vi "Interface_main.vi"() -> ()   [LabVIEW 2013]
uses:
  Controls/Steering Inputs.ctl
  Controls/Intuitive Steering.ctl
  Controls/Steering Mode.ctl
  Controls/SpaceMouse_Parameters.ctl
  Controls/SpaceMouse_Buttons.ctl
  Controls/Fin Arrangement.ctl
  Controls/Swimbladder Tuning Parameters.ctl
  Controls/Sensors State.ctl
  Controls/Sepios General Parameters.ctl
  Controls/Fin Status.ctl
  myRIO/Sensors/IMU/IMU_Data_Type_Def.ctl
  Controls/Advanced Swimbladder Indicators.ctl
  Controls/Battery_level.ctl
  Controls/Sepios_status.ctl
  Controls/Attitude Controllers Parameters.ctl
  Controls/EKF_Settings.ctl
  Controls/Estimated Position.ctl
  Controls/Individual Steering.ctl
  Controls/IndividualSteering_f(x)_enum.ctl
  Controls/Flow/Flow_Velocity.ctl
  Controls/Flow/Flow_Acceleration.ctl
  Controls/Flow/Flow_Number_dig.ctl
  Controls/Individual Steering Configurations.ctl
  Controls/Flow/Flow_Throttle.ctl
  Controls/Flow/Velocity Controllers Parameters.ctl
  Controls/Flow/Flow_Variables.ctl
  Controls/SpaceMouse_FilteredInput.ctl
  Controls/SpaceMouse_RawInput.ctl
  Controls/Servo Position.ctl
  <vilib>/Utility/xml.llb/Write to XML File(string).vi
  <vilib>/Utility/xml.llb/Read From XML File(string).vi
  myRIO/Sensors/IMU/Attitude display/Bsp. Attitude Display/lv-attitudecontrol.lvlib
panel:
  out "Fin Status":T1=[16777215, 16777215, 16777215, 16777215]
  in  "Fin Arrangement":T2={"Fin0"=0, "Fin3"=3, "Fin1"=1, "Fin2"=2} {"Fin2" items=["0", "1", "2", "3"]; "Fin1" items=["0", "1", "2", "3"]; "Fin3" items=["0", "1", "2", "3"]; "Fin0" items=["0", "1", "2", "3"]}
  out "Main_Current [A]":dbl(knob) scale=0.0..50.0
  out "tooDeep":bool
  out "LEAKAGE":bool
  out "Depth [m]":cluster{dbl, dbl, dbl}(slide)={0.0, 0.0, 3.5} scale format="%#_3g"
  in  "Steering Mode":T3
  in  "Tab Control":T4(tab)
  in  "Attitude Sepios":refnum<vi>(3d-picture)
  out "Battery_level":T5=86.537845 scale=0.0..100.0
  in  "Full Battery?":bool
  out "Time left [min]":dbl=inf
  out "Sepios_Status":T6
  in  "Desired Attitude":refnum<vi>(3d-picture)
  in  "Attitude Control On":bool
  in  "Auto stable when idle":bool
  out "Brake":bool
  in  "STOP_Steering":bool
  in  "Intuitive Steering User Control":T7={"Frequency (Hz):"=0.7, "Max. Amplitude (°):"=25.0, "Phase Shift (/Pi):"=0.25, "Flap (°):"=90.0, "Flap Saturation:"=0.7} {"Flap Saturation:" min=0.0 max=1.0 step=0.1; "Flap (°):" min=0.0 max=90.0 step=5.0; "Phase Shift (/Pi):" min=-1.0 max=1.0 step=0.1; "Max. Amplitude (°):" min=0.0 max=135.0 step=1.0; "Frequency (Hz):" min=0.0 max=2.0 step=0.1}
  out "Bottom Fin (2)":cluster{dbl, dbl, "FinPositions":dbl[]}(graph)={0.0, 1.0, "FinPositions"=[0.0, 0.0, 0.0, 0.0, 0.0, 0.0, 0.0, 0.0, 0.0]}
  out "Right Fin (1)":cluster{dbl, dbl, "FinPositions":dbl[]}(graph)={0.0, 1.0, "FinPositions"=[0.0, 0.0, 0.0, 0.0, 0.0, 0.0, 0.0, 0.0, 0.0]}
  out "Left Fin (3)":cluster{dbl, dbl, "FinPositions":dbl[]}(graph)={0.0, 1.0, "FinPositions"=[0.0, 0.0, 0.0, 0.0, 0.0, 0.0, 0.0, 0.0, 0.0]}
  out "Top Fin (0)":cluster{dbl, dbl, "FinPositions":dbl[]}(graph)={0.0, 1.0, "FinPositions"=[0.0, 0.0, 0.0, 0.0, 0.0, 0.0, 0.0, 0.0, 0.0]}
  in  "IndividualSteering_f(x)":T8
  in  "Individual Steering":T9=[{"Fin Parameters"=[{"Amplitude"=20.0, "Phase Shift"=0.25, "Zero Position"=0.0}, {"Amplitude"=20.0, "Phase Shift"=0.25, "Zero Position"=0.0}, {"Amplitude"=20.0, "Phase Shift"=0.25, "Zero Position"=0.0}, {"Amplitude"=20.0, "Phase Shift"=0.25, "Zero Position"=0.0}, {"Amplitude"=20.0, "Phase Shift"=0.25, "Zero Position"=0.0}, {"Amplitude"=20.0, "Phase Shift"=0.25, "Zero Position"=0.0}, {"Amplitude"=20.0, "Phase Shift"=0.25, "Zero Position"=0.0}, {"Amplitude"=20.0, "Phase Shift"=0.25, "Zero Position"=0.0}, {"Amplitude"=20.0, "Phase Shift"=0.25, "Zero Position"=0.0}], "Frequency\n& Direction"=0.7, "General A, PS, ZP"={"Amplitude"=20.0, "Phase Shift"=0.25, "Zero Position"=0.0}}, {"Fin Parameters"=[{"Amplitude"=20.0, "Phase Shift"=0.25, "Zero Position"=0.0}, {"Amplitude"=20.0, "Phase Shift"=0.25, "Zero Position"=0.0}, {"Amplitude"=20.0, "Phase Shift"=0.25, "Zero Position"=0.0}, {"Amplitude"=20.0, "Phase Shift"=0.25, "Zero Position"=0.0}, {"Amplitude"=20.0, "Phase Shift"=0.25, "Zero Position"=0.0}, {"Amplitude"=20.0, "Phase Shift"=0.25, "Zero Position"=0.0}, {"Amplitude"=20.0, "Phase Shift"=0.25, "Zero Position"=0.0}, {"Amplitude"=20.0, "Phase Shift"=0.25, "Zero Position"=0.0}, {"Amplitude"=20.0, "Phase Shift"=0.25, "Zero Position"=0.0}], "Frequency\n& Direction"=0.7, "General A, PS, ZP"={"Amplitude"=20.0, "Phase Shift"=0.25, "Zero Position"=0.0}}, {"Fin Parameters"=[{"Amplitude"=20.0, "Phase Shift"=0.25, "Zero Position"=0.0}, {"Amplitude"=20.0, "Phase Shift"=0.25, "Zero Position"=0.0}, {"Amplitude"=20.0, "Phase Shift"=0.25, "Zero Position"=0.0}, {"Amplitude"=20.0, "Phase Shift"=0.25, "Zero Position"=0.0}, {"Amplitude"=20.0, "Phase Shift"=0.25, "Zero Position"=0.0}, {"Amplitude"=20.0, "Phase Shift"=0.25, "Zero Position"=0.0}, {"Amplitude"=20.0, "Phase Shift"=0.25, "Zero Position"=0.0}, {"Amplitude"=20.0, "Phase Shift"=0.25, "Zero Position"=0.0}, {"Amplitude"=20.0, "Phase Shift"=0.25, "Zero Position"=0.0}], "Frequency\n& Direction"=0.7, "General A, PS, ZP"={"Amplitude"=20.0, "Phase Shift"=0.25, "Zero Position"=0.0}}, {"Fin Parameters"=[{"Amplitude"=20.0, "Phase Shift"=0.25, "Zero Position"=0.0}, {"Amplitude"=20.0, "Phase Shift"=0.25, "Zero Position"=0.0}, {"Amplitude"=20.0, "Phase Shift"=0.25, "Zero Position"=0.0}, {"Amplitude"=20.0, "Phase Shift"=0.25, "Zero Position"=0.0}, {"Amplitude"=20.0, "Phase Shift"=0.25, "Zero Position"=0.0}, {"Amplitude"=20.0, "Phase Shift"=0.25, "Zero Position"=0.0}, {"Amplitude"=20.0, "Phase Shift"=0.25, "Zero Position"=0.0}, {"Amplitude"=20.0, "Phase Shift"=0.25, "Zero Position"=0.0}, {"Amplitude"=20.0, "Phase Shift"=0.25, "Zero Position"=0.0}], "Frequency\n& Direction"=0.7, "General A, PS, ZP"={"Amplitude"=20.0, "Phase Shift"=0.25, "Zero Position"=0.0}}] {"General A, PS, ZP"."Zero Position" min=-135.0 max=135.0 step=1.0; "General A, PS, ZP"."Phase Shift" min=-1.0 max=1.0 step=0.1; "General A, PS, ZP"."Amplitude" min=0.0 max=135.0 step=1.0; "Frequency\n& Direction" min=-2.0 max=2.0 step=0.1; "Fin Parameters"."Zero Position" min=-135.0 max=135.0 step=1.0; "Fin Parameters"."Phase Shift" min=-1.0 max=1.0 step=0.1; "Fin Parameters"."Amplitude" min=0.0 max=135.0 step=1.0}
  in  "Individual Steering Configurations":T10
  in  "Max Depth":dbl=3.5 max=10.0 step=0.25
  in  "Depth Desired [m]":dbl max=10.0 step=0.1
  in  "STOP_Swimbladder":bool=TRUE
  in  "Swimbladder Tuning Parameters":T11={"Excessive_Depth_Deviation_Trigger"=0.4, "Neutral Buoancy_x"=0.2, "Ti_Depth_Control"=1e-05, "kp_Depth_Control"=0.3, "Integrator enabled range Depth"=0.15, "Integrator_enable_Range_Motor"=0.03, "kp_Motor"=150.0, "Ti_Motor"=1.72e-05} {"Ti_Motor" min=0.0 step=0.0001; "kp_Motor" min=0.0 max=20.0 step=0.01; "Integrator_enable_Range_Motor" min=0.0 step=0.01}
  out "Advanced Swimbladder Indicators":T12={"P_ref [Pa]"=100000.0, "X_Actual [m]"=0.0, "Motor Current[A]"=0.0} {"Motor Current[A]" scale=0.0..3.0}
  out "X_Desired":dbl
  out "X_Actual [m]":dbl(slide) scale=0.0..0.42
  out "SB_Piston_Stuck":bool
  in  "EKF_Settings":T13={"Gravity constant"=-9.808205458883663, "Filter Version"=enum."IMU, Pressure, Compass", "Initial Biases"={"Gyro_Bias_nit_x"=0.00198, "Gyro_Bias_init_y"=0.0053, "Gyro_Bias_init_z"=0.0009, "Acc_Bias_init_x"=0.0, "Acc_Bias_init_y"=0.0, "Acc_Bias_init_z"=0.0}, "Use Compass on initialisation"=TRUE, "Initial Biases Covariances"={"Initial_covariance_Gyro_Bias"=0.0014, "Initial_covariance_Acc_Bias"=0.2}, "Magnetic-Field-Vector [utesla]"={"Magf_N_x"=21.565, "Magf_N_y"=0.6833, "Magf_N_z"=42.6149}, "IMU_Sigmas"={"Sigma_w"=0.00033937, "Sigma_wb"=3.8785e-05, "Sigma_a"=0.02, "Sigma_ab"=0.03, "Sigma_m"=1000.0}, "Measurement Sigmas"={"Sigma_v"=500.0, "Sigma_depth"=0.2}}
  out "Estimated Position":T14
  in  "Attitude_Increase_Speed [rad]":dbl=0.01 format="%#_13g"
  in  "Attitude Controllers Parameters":T15={"ARW on"={"Phi"=TRUE, "Theta"=TRUE, "Psi"=TRUE}, "kp"={"kp Phi"=4.0, "kp Theta"=8.0, "kp Psi"=5.0}, "Ti"={"Ti Phi"=0.2, "Ti Theta"=0.01, "Ti Psi"=0.01}, "Integrator enabled range [rad      "={"I_E Phi"=0.4, "I_E Theta"=0.2, "I_E Psi"=0.2}}
  in  "Intuitive Steering Attitude Control":T7={"Frequency (Hz):"=0.8, "Max. Amplitude (°):"=40.0, "Phase Shift (/Pi):"=0.25, "Flap (°):"=20.0, "Flap Saturation:"=0.7} {"Flap Saturation:" min=0.0 max=1.0 step=0.1; "Flap (°):" min=0.0 max=90.0 step=5.0; "Phase Shift (/Pi):" min=-1.0 max=1.0 step=0.1; "Max. Amplitude (°):" min=0.0 max=135.0 step=1.0; "Frequency (Hz):" min=0.0 max=2.0 step=0.1}
  in  "Tab Control 2":T16(tab)
  out "Speed":dbl(graph)
  in  "Throttle":T17 scale=0.0..0.6
  in  "Velocity Control on":bool
  out "Flow_LED":bool
  out "Value":T18 format="%.2g"
  out "Acceleration [m/s2]":T19 scale=0.0..5.0 scale format="%.1g"
  out "Speed [m/s]":T20 scale=0.0..2.8 scale format="%.1g"
  out "Flow_variables":T21
  in  "Velocity Controllers Parameters":T22
  out "spiderplot":picture
  in  "SpaceMouse_Refresh":bool
  in  "SpaceMouse_EnableInputs":T23={"X"=TRUE, "Y"=TRUE, "Z"=TRUE, "phi"=TRUE, "theta"=TRUE, "psi"=TRUE, "All Inputs"=TRUE}
  out "Raw Input":T24(graph)
  out "Filtered Input":T25(graph)
  out "SpaceMouse_Buttons":T26={"Idle"=TRUE, "Button Right"=FALSE, "Button Left"=FALSE}
  in  "SpaceMouse_Parameters":T27={"Lowpass Filter Cutoff Frequency"=10.0, "Idle Threshold"=50.0, "Deadzone"=15000.0, "Filter Sample Size"=25, "FilterOff"=FALSE, "IntegratorOff"=FALSE} {"Filter Sample Size" min=0 max=100 step=1; "Deadzone" min=0.0 max=32767.0 step=100.0; "Idle Threshold" min=0.0 max=32767.0 step=10.0; "Lowpass Filter Cutoff Frequency" min=0.0 max=10.0 step=0.1}
  in  "Sensors State":T28={"Leakage-Sensor_enabled"=TRUE, "IMU_enabled"=TRUE, "Swimbladder Fill-State-Sensor_enabled"=TRUE, "Flow-Sensor_enabled"=FALSE, "Depth-Sensor_enabled"=TRUE, "Current-Sensor_enabled"=TRUE, "Calibrate Depth"=FALSE, "SB_Piston_Stuck_Detect_enabled"=FALSE, "Check_too_Deep_enabled"=TRUE}
  out "IMU_Data_simple":T29
  out "Avoidance":bool
  out "Laser Detected":bool
  in  "Collision\nAvoidance":bool
  in  "Laser":bool
  in  "Camera":bool=TRUE
  in  "Overlay":bool
  in  "Collision\nDetection":bool
  out "Collision":bool
  in  "STOP_LiveStream":bool=TRUE
  out "Live Stream":T30(plugin-control)
  in  "Path":path=path "C:/Users/Antoine/Desktop"
  in  "AVI Name":string="test"
  in  "Record Button":bool
  in  "Pic Name":string="test"
  in  "Picture Button":bool
  out "Incident Angle [°]":dbl
  out "Perp. Distance [m]":dbl
  out "Distance [m]":dbl
  in  "Load Parameters from File":bool
  in  "Save Parameters to File":bool
  in  "Sepios General Parameters":T31={"Sensors-Settings"={"Water density [kg/m3]"=1000.0, "SB_parameters"={"x0"=0.0, "U_full"=0.695, "U_empty"=3.67}}, "Startup"={"Enable Swimbladder"=FALSE}, "Default Configuration File"=path ""}
  out "error out":errorcluster={"status"=FALSE, "code"=-2220, "source"=""}
  in  "Create New Log":bool
  in  "group name":string="IMU, DepthSensor,CurrentSensor"
  in  "Period [ms]":i64=10
  in  "TDMS: file name":string="sepiosLOG" caption="default name"
  in  "channel name(s)":string[](array[string])=["X_Gyro", "Y_Gyro", "Z_Gyro", "X_Accl", "Y_Accl", "Z_Accl", "X_Magn", "Y_Magn", "Z_Magn", "IMU_Temp", "IMU_Barom", "Depth", "Current"]
  out "Sampling Frequ.\ntoo LOW":bool
  in  "Viewer_enable":bool
  in  "Exit":bool
  in  "Standby":bool=TRUE
  in  "User Steering Inputs":T32 {"psi" min=-1.0 max=1.0 step=0.1 scale=-1.0..1.0; "theta" min=-1.0 max=1.0 step=0.1 scale=-1.0..1.0; "phi" min=-1.0 max=1.0 step=0.1 scale=-1.0..1.0; "Z" min=-1.0 max=1.0 step=0.1 scale=-1.0..1.0; "Y" min=-1.0 max=1.0 step=0.1 scale=-1.0..1.0; "X" min=-1.0 max=1.0 step=0.1 scale=-1.0..1.0}
  # "Amplitude"
  # "Phase Shift"
  # "Zero Position"
  # "positive means down"
  # "In order to have velocity control turn off collision detection and attitude control:"
  # "Here deflection spider graphs will be displayed"
  # "Calibrate Depth\nButton??"
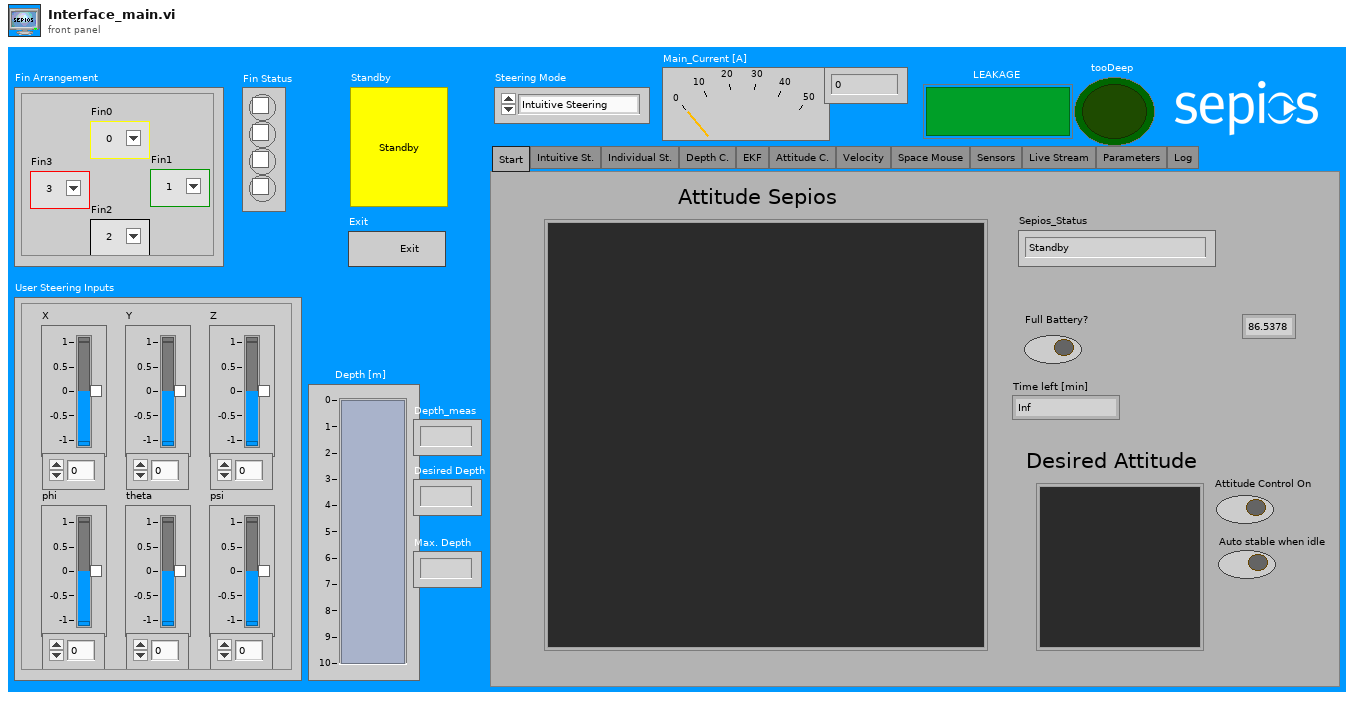
[diagram p1: front panel]
types:
  T1 = typedef "Fin Status.ctl" = u32[]
  T2 = typedef "Fin Arrangement.ctl" = cluster{"Fin0":u8, "Fin3":u8, "Fin1":u8, "Fin2":u8}
  T3 = typedef "Steering Mode.ctl" = enum16{"Intuitive Steering", "Control Allocation", "Individually"}
  T4 = enum32{"Start", "Intuitive St.", "Individual St.", "Depth C.", "EKF", "Attitude C.", "Velocity", "Space Mouse", "Sensors", "Live Stream", "Parameters", "Log"}
  T5 = typedef "Battery_level.ctl" = dbl
  T6 = typedef "Sepios_status.ctl" = enum16{"Standby", "Running", "Filming", "Error"}
  T7 = typedef "Intuitive Steering.ctl" = cluster{"Frequency (Hz):":dbl, "Max. Amplitude (°):":dbl, "Phase Shift (/Pi):":dbl, "Flap (°):":dbl, "Flap Saturation:":dbl}
  T8 = typedef "IndividualSteering_f(x)_enum.ctl" = enum16{"sin(x)", "cuttlefish sine", "cuttlefish triangle", "triangle"}
  T9 = typedef "Individual Steering.ctl" = cluster{"Fin Parameters":cluster{"Amplitude":dbl, "Phase Shift":dbl, "Zero Position":dbl}[], "Frequency\n& Direction":dbl, "General A, PS, ZP":cluster{"Amplitude":dbl, "Phase Shift":dbl, "Zero Position":dbl}}[]
  T10 = typedef "Individual Steering Configurations.ctl" = cluster{"Standard":bool, "Left Curve":bool, "Screw":bool, "Inclined":bool, "Looping":bool, "Cuttle":bool}
  T11 = typedef "Swimbladder Tuning Parameters.ctl" = cluster{"Excessive_Depth_Deviation_Trigger":dbl, "Neutral Buoancy_x":dbl, "Ti_Depth_Control":dbl, "kp_Depth_Control":dbl, "Integrator enabled range Depth":dbl, "Integrator_enable_Range_Motor":dbl, "kp_Motor":dbl, "Ti_Motor":dbl}
  T12 = typedef "Advanced Swimbladder Indicators.ctl" = cluster{"P_ref [Pa]":dbl, "X_Actual [m]":dbl, "Motor Current[A]":dbl}
  T13 = typedef "EKF_Settings.ctl" = cluster{"Gravity constant":dbl, "Filter Version":enum16{"IMU Only", "IMU & Pressure", "IMU, Pressure, Compass"}, "Initial Biases":cluster{"Gyro_Bias_nit_x":dbl, "Gyro_Bias_init_y":dbl, "Gyro_Bias_init_z":dbl, "Acc_Bias_init_x":dbl, "Acc_Bias_init_y":dbl, "Acc_Bias_init_z":dbl}, "Use Compass on initialisation":bool, "Initial Biases Covariances":cluster{"Initial_covariance_Gyro_Bias":dbl, "Initial_covariance_Acc_Bias":dbl}, "Magnetic-Field-Vector [utesla]":cluster{"Magf_N_x":dbl, "Magf_N_y":dbl, "Magf_N_z":dbl}, "IMU_Sigmas":cluster{"Sigma_w":dbl, "Sigma_wb":dbl, "Sigma_a":dbl, "Sigma_ab":dbl, "Sigma_m":dbl}, "Measurement Sigmas":cluster{"Sigma_v":dbl, "Sigma_depth":dbl}}
  T14 = typedef "Estimated Position.ctl" = cluster{"X":dbl, "Y":dbl, "Z":dbl, "V_X":dbl, "V_Y":dbl, "V_Z":dbl}
  T15 = typedef "Attitude Controllers Parameters.ctl" = cluster{"ARW on":cluster{"Phi":bool, "Theta":bool, "Psi":bool}, "kp":cluster{"kp Phi":dbl, "kp Theta":dbl, "kp Psi":dbl}, "Ti":cluster{"Ti Phi":dbl, "Ti Theta":dbl, "Ti Psi":dbl}, "Integrator enabled range [rad      ":cluster{"I_E Phi":dbl, "I_E Theta":dbl, "I_E Psi":dbl}}
  T16 = enum32{"Speedometer", "Control Parameters and Advanved Indicators"}
  T17 = typedef "Flow_Throttle.ctl" = dbl
  T18 = typedef "Flow_Number_dig.ctl" = dbl
  T19 = typedef "Flow_Acceleration.ctl" = sgl
  T20 = typedef "Flow_Velocity.ctl" = sgl
  T21 = typedef "Flow_Variables.ctl" = cluster{"u_Body":dbl, "v_Body":dbl, "w_Body":dbl, "omega_x_Body":dbl, "omega_z_Body":dbl, "omega_y_Body":dbl}
  T22 = typedef "Velocity Controllers Parameters.ctl" = cluster{"ARW on":cluster{"u":bool, "v":bool, "w":bool}, "kp":cluster{"kp_u":dbl, "kp_v":dbl, "kp_w":dbl}, "Ti":cluster{"Ti_u":dbl, "Ti_v":dbl, "Ti_w":dbl}, "Integrator enabled range [m/s]      ":cluster{"I_E_u":dbl, "I_E_v":dbl, "I_E_w":dbl}}
  T23 = cluster{"X":bool, "Y":bool, "Z":bool, "phi":bool, "theta":bool, "psi":bool, "All Inputs":bool}
  T24 = cluster{"X":i32, "Y":i32, "Z":i32, "phi":i32, "theta":i32, "psi":i32}
  T25 = cluster{"X":dbl, "Y":dbl, "Z":dbl, "phi":dbl, "theta":dbl, "psi":dbl}
  T26 = typedef "SpaceMouse_Buttons.ctl" = cluster{"Idle":bool, "Button Right":bool, "Button Left":bool}
  T27 = typedef "SpaceMouse_Parameters.ctl" = cluster{"Lowpass Filter Cutoff Frequency":dbl, "Idle Threshold":dbl, "Deadzone":dbl, "Filter Sample Size":i32, "FilterOff":bool, "IntegratorOff":bool}
  T28 = typedef "Sensors State.ctl" = cluster{"Leakage-Sensor_enabled":bool, "IMU_enabled":bool, "Swimbladder Fill-State-Sensor_enabled":bool, "Flow-Sensor_enabled":bool, "Depth-Sensor_enabled":bool, "Current-Sensor_enabled":bool, "Calibrate Depth":bool, "SB_Piston_Stuck_Detect_enabled":bool, "Check_too_Deep_enabled":bool}
  T29 = typedef "IMU_Data_Type_Def.ctl" = cluster{timestamp, "X_Gyro_Out":dbl, "Y_Gyro_Out":dbl, "Z_Gyro_Out":dbl, "X_Accl_Out":dbl, "Y_Accl_Out":dbl, "Z_Accl_Out":dbl, "X_Magn_Out":dbl, "Y_Magn_Out":dbl, "Z_Magn_Out":dbl, "Temp_Out":dbl, "Barom_Out":dbl}
  T30 = typedef "IMAQ Image.ctl" = refnum<image>
  T31 = typedef "Sepios General Parameters.ctl" = cluster{"Sensors-Settings":cluster{"Water density [kg/m3]":dbl, "SB_parameters":cluster{"x0":dbl, "U_full":dbl, "U_empty":dbl}}, "Startup":cluster{"Enable Swimbladder":bool}, "Default Configuration File":path}
  T32 = typedef "Steering Inputs.ctl" = cluster{"X":dbl, "Y":dbl, "Z":dbl, "phi":dbl, "theta":dbl, "psi":dbl}
  T33 = cluster{"New attitude phi":dbl, "New attitude theta":dbl, "New attitude psi":dbl}
  T34 = cluster{"Rows Per Strip":i32, "Photometric":i32, "Compression Type":i32}
  T35 = typedef "lv-attitudecontrol.lvlib/AttitudeHandle.ctl" = cluster{"First Scene Object":refnum<vi>, "Drum":refnum<vi>, "Window":refnum<vi>, "Dial":refnum<vi>, "Scene Graph":refnum<vi>, "Last Drum Pitch":dbl, "Last Drum Roll ":dbl, "Last Dial Roll":dbl}
  T36 = typedef "SpaceMouse_FilteredInput.ctl" = cluster{"X":dbl, "Y":dbl, "Z":dbl, "phi":dbl, "theta":dbl, "psi":dbl}
  T37 = typedef "SpaceMouse_RawInput.ctl" = cluster{"X":i32, "Y":i32, "Z":i32, "phi":i32, "theta":i32, "psi":i32}
  T38 = cluster{"All Inputs":bool, "All Inputs":bool, "All Inputs":bool, "All Inputs":bool, "All Inputs":bool, "All Inputs":bool, "All Inputs":bool}
  T39 = typedef "IMAQ AVI2 Refnum.ctl" = refnum<k20>
  T40 = typedef "Servo Position.ctl" = dbl[][]
  T41 = cluster{"u_Body":dbl, "v_Body":dbl, "w_Body":dbl, "omega_x_Body":dbl, "omega_z_Body":dbl, "omega_y_Body":dbl}
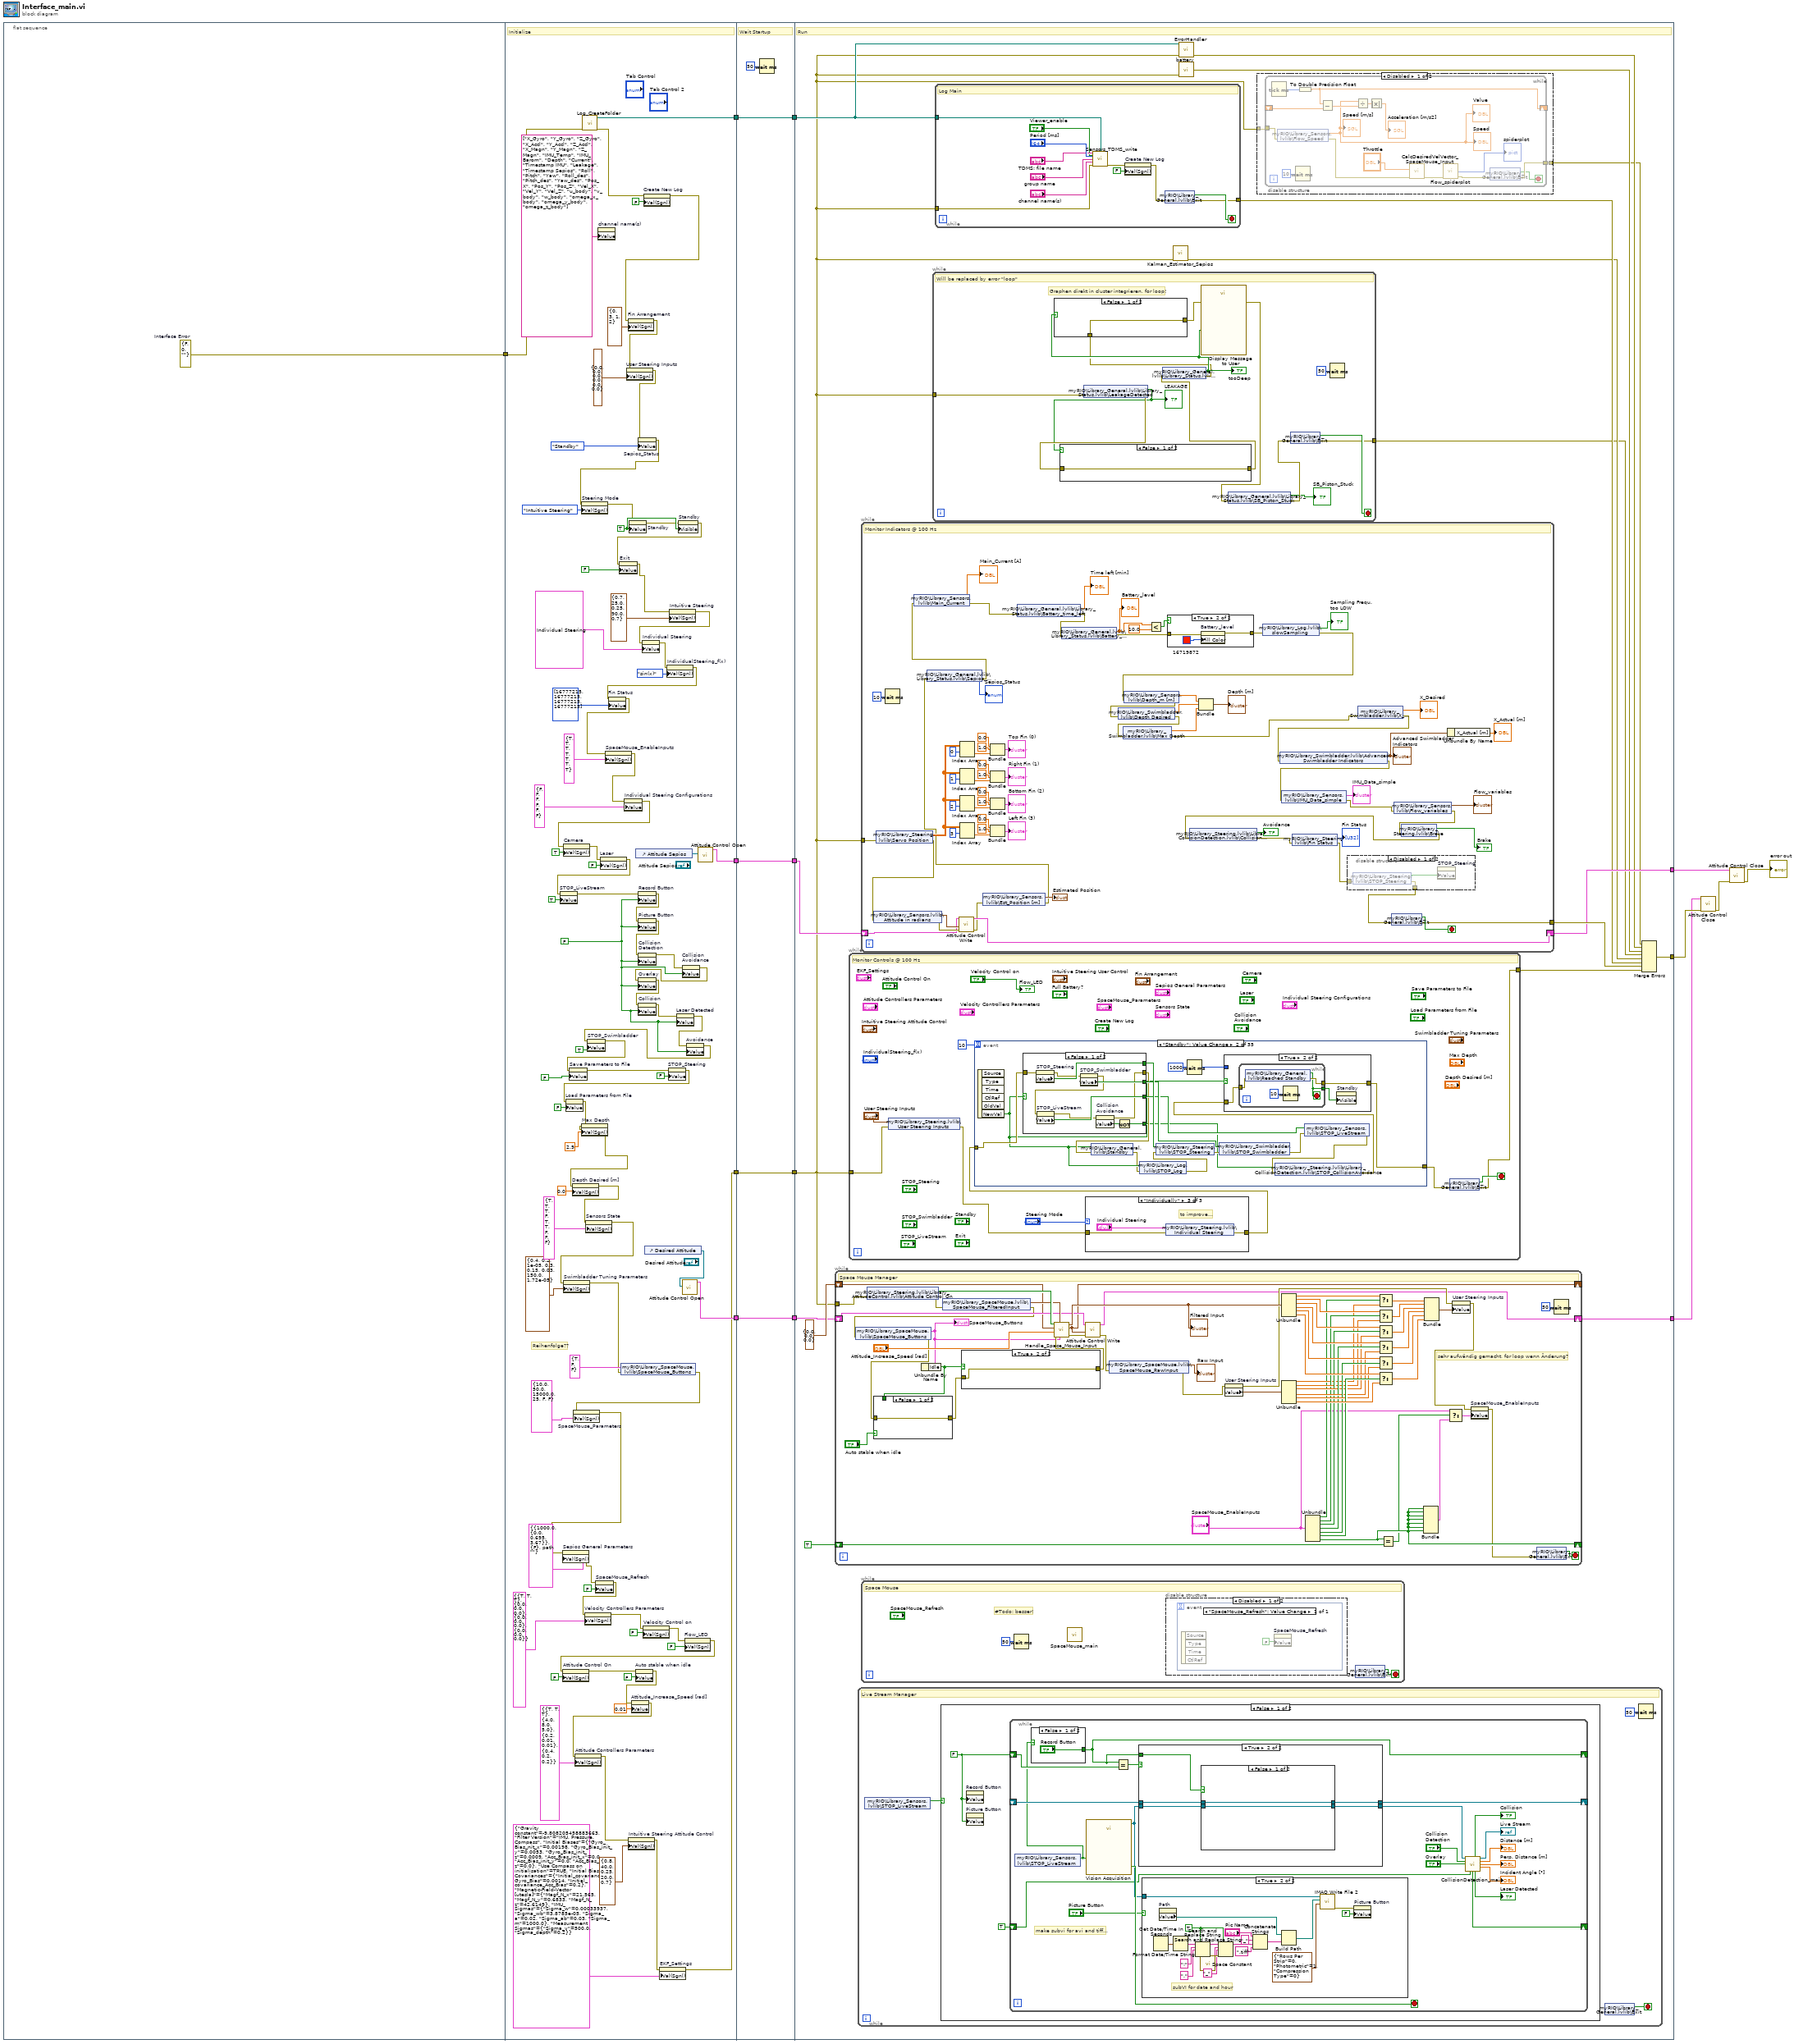
[diagram p0: block diagram]
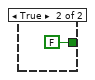
[diagram p4: hidden frame]
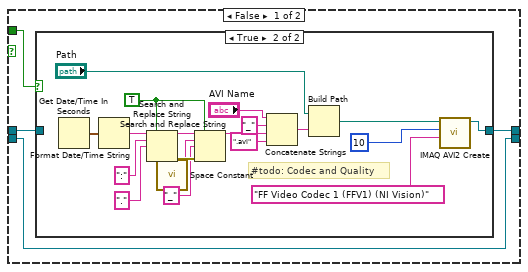
[diagram p5: hidden frame]
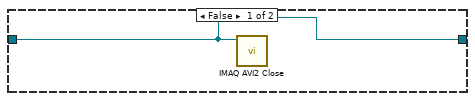
[diagram p6: hidden frame]
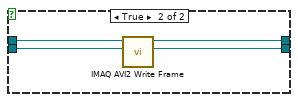
[diagram p7: hidden frame]
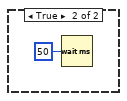
[diagram p8: hidden frame]
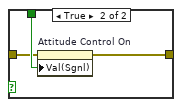
[diagram p10: hidden frame]
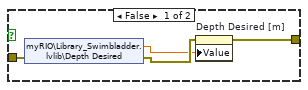
[diagram p11: hidden frame]
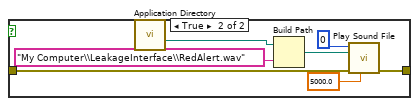
[diagram p12: hidden frame]
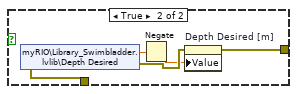
[diagram p13: hidden frame]
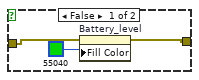
[diagram p15: hidden frame]
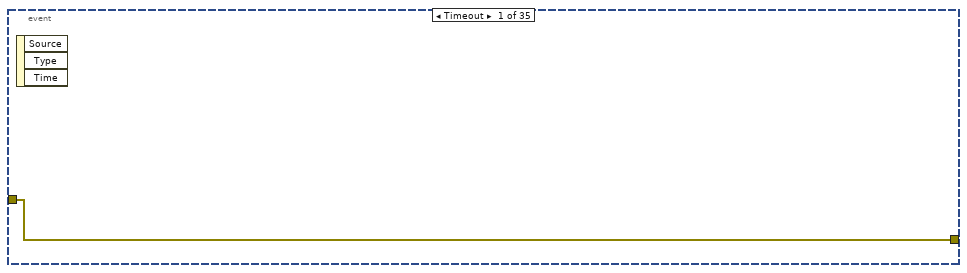
[diagram p18: hidden frame]
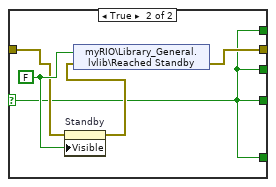
[diagram p20: hidden frame]
diagram:
  n1 = flat-sequence {
    tunnel: [w15] -> w14
    tunnel: w14 -> [w49]
    tunnel: [w51] -> w12
    tunnel: [w75] -> w10
    tunnel: [w69] -> w3
    tunnel: [w48] -> w1
    tunnel: [w111] -> w13
    tunnel: w12 -> [w111]
    tunnel: [w110] -> w11
    tunnel: w10 -> [w110]
    tunnel: [w109] -> w4
    tunnel: w3 -> [w109]
    tunnel: [w108] -> w2
    tunnel: w1 -> [w108]
    tunnel: [w127] -> w7
    tunnel: w13 -> [w114]
    tunnel: w11 -> [w121]
    tunnel: [w126] -> w9
    tunnel: [w120] -> w5
    tunnel: w4 -> [w118]
    tunnel: w2 -> [w115]
    frame #0 {
      w15 = errorcluster {"status"=FALSE, "code"=0, "source"=""}  # Interface Error
    }
    frame #1 {
      w16 = FALSE ("Collision\nDetection")
      w74 = TRUE ("Running")
      # "Reihenfolge??"
      # "Initialize"
      n2 = call "Log_CreateFolder.vi"("error in (no error)"=w49) -> ("error out"=w38:errorcluster, "created path"=w48:path)  [unwired: 9 in]
      n3 = property on="channel name(s)" class="Arr (strict)"("Value"=string[] ["X_Gyro", "Y_Gyro", "Z_Gyro", "X_Accl", "Y_Accl", "Z_Accl", "X_Magn", "Y_Magn", "Z_Magn", "IMU_Temp", "IMU_Barom", "Depth", "Current", "Timestamp IMU", "Leakage", "Timestamp Sepios", "Roll", "Pitch", "Yaw", "Roll_des", "Pitch_des", "Yaw_des", "Pos_X", "Pos_Y", "Pos_Z", "Vel_X", "Vel_Y", "Vel_Z", "u_body", "v_body", "w_body", "omega_x_body", "omega_y_body", "omega_z_body"] ("channel name(s)")) -> ()  [unwired: 2 in, 2 out]
      n4 = control-ref of="Attitude Sepios"() -> (w76:refnum<vi>)
      n5 = property on="Create New Log" class="Bool (strict)"(error in=w38, "Val(Sgnl)"=FALSE ("Value (Signaling)")) -> (error out=w37:errorcluster)  [unwired: 1 in, 1 out]
      n6 = property on="Fin Arrangement" class="Clust (strict)"(error in=w37, "Val(Sgnl)"=T2 {"Fin0"=0, "Fin3"=3, "Fin1"=1, "Fin2"=2} ("Fin Arrangement")) -> (error out=w96:errorcluster)  [unwired: 1 in, 1 out]
      n7 = property on="User Steering Inputs" class="Clust (strict)"(error in=w96, "Val(Sgnl)"=T32 {"X"=0.0, "Y"=0.0, "Z"=0.0, "phi"=0.0, "theta"=0.0, "psi"=0.0} ("Steering Inputs")) -> (error out=w70:errorcluster)  [unwired: 1 in, 1 out]
      n8 = property on="Sepios_Status" class="Enum (strict)"(error in=w70, "Value"=Sepios_status."Standby" ("Sepios_Status")) -> (error out=w42:errorcluster)  [unwired: 1 in, 1 out]
      n9 = property on="Steering Mode" class="Enum (strict)"(error in=w42, "Val(Sgnl)"=Steering_Mode."Intuitive Steering" ("Value (Signaling)")) -> (error out=w41:errorcluster)  [unwired: 1 in, 1 out]
      n10 = property on="Standby" class="Bool (strict)"(error in=w41, "Value"=w74) -> (error out=w73:errorcluster)  [unwired: 1 in, 1 out]
      n11 = control-ref of="Desired Attitude"() -> (w68:refnum<vi>)
      n12 = property on="Standby" class="Bool (strict)"(error in=w73, "Visible"=w74) -> (error out=w72:errorcluster)  [unwired: 1 in, 1 out]
      n13 = property on="Exit" class="Bool (strict)"(error in=w72, "Value"=FALSE ("Exit")) -> (error out=w59:errorcluster)  [unwired: 1 in, 1 out]
      n14 = property on="Intuitive Steering" class="Clust (strict)"(error in=w59, "Val(Sgnl)"=T7 {"Frequency (Hz):"=0.7, "Max. Amplitude (°):"=25.0, "Phase Shift (/Pi):"=0.25, "Flap (°):"=90.0, "Flap Saturation:"=0.7} ("Value (Signaling)")) -> (error out=w35:errorcluster)  [unwired: 1 in, 1 out]
      n15 = property on="Individual Steering" class="Arr (strict)"(error in=w35, "Value"=T9 [{"Fin Parameters"=[{"Amplitude"=20.0, "Phase Shift"=0.25, "Zero Position"=0.0}, {"Amplitude"=20.0, "Phase Shift"=0.25, "Zero Position"=0.0}, {"Amplitude"=20.0, "Phase Shift"=0.25, "Zero Position"=0.0}, {"Amplitude"=20.0, "Phase Shift"=0.25, "Zero Position"=0.0}, {"Amplitude"=20.0, "Phase Shift"=0.25, "Zero Position"=0.0}, {"Amplitude"=20.0, "Phase Shift"=0.25, "Zero Position"=0.0}, {"Amplitude"=20.0, "Phase Shift"=0.25, "Zero Position"=0.0}, {"Amplitude"=20.0, "Phase Shift"=0.25, "Zero Position"=0.0}, {"Amplitude"=20.0, "Phase Shift"=0.25, "Zero Position"=0.0}], "Frequency\n& Direction"=0.7, "General A, PS, ZP"={"Amplitude"=20.0, "Phase Shift"=0.25, "Zero Position"=0.0}}, {"Fin Parameters"=[{"Amplitude"=20.0, "Phase Shift"=0.25, "Zero Position"=0.0}, {"Amplitude"=20.0, "Phase Shift"=0.25, "Zero Position"=0.0}, {"Amplitude"=20.0, "Phase Shift"=0.25, "Zero Position"=0.0}, {"Amplitude"=20.0, "Phase Shift"=0.25, "Zero Position"=0.0}, {"Amplitude"=20.0, "Phase Shift"=0.25, "Zero Position"=0.0}, {"Amplitude"=20.0, "Phase Shift"=0.25, "Zero Position"=0.0}, {"Amplitude"=20.0, "Phase Shift"=0.25, "Zero Position"=0.0}, {"Amplitude"=20.0, "Phase Shift"=0.25, "Zero Position"=0.0}, {"Amplitude"=20.0, "Phase Shift"=0.25, "Zero Position"=0.0}], "Frequency\n& Direction"=0.7, "General A, PS, ZP"={"Amplitude"=20.0, "Phase Shift"=0.25, "Zero Position"=0.0}}, {"Fin Parameters"=[{"Amplitude"=20.0, "Phase Shift"=0.25, "Zero Position"=0.0}, {"Amplitude"=20.0, "Phase Shift"=0.25, "Zero Position"=0.0}, {"Amplitude"=20.0, "Phase Shift"=0.25, "Zero Position"=0.0}, {"Amplitude"=20.0, "Phase Shift"=0.25, "Zero Position"=0.0}, {"Amplitude"=20.0, "Phase Shift"=0.25, "Zero Position"=0.0}, {"Amplitude"=20.0, "Phase Shift"=0.25, "Zero Position"=0.0}, {"Amplitude"=20.0, "Phase Shift"=0.25, "Zero Position"=0.0}, {"Amplitude"=20.0, "Phase Shift"=0.25, "Zero Position"=0.0}, {"Amplitude"=20.0, "Phase Shift"=0.25, "Zero Position"=0.0}], "Frequency\n& Direction"=0.7, "General A, PS, ZP"={"Amplitude"=20.0, "Phase Shift"=0.25, "Zero Position"=0.0}}, {"Fin Parameters"=[{"Amplitude"=20.0, "Phase Shift"=0.25, "Zero Position"=0.0}, {"Amplitude"=20.0, "Phase Shift"=0.25, "Zero Position"=0.0}, {"Amplitude"=20.0, "Phase Shift"=0.25, "Zero Position"=0.0}, {"Amplitude"=20.0, "Phase Shift"=0.25, "Zero Position"=0.0}, {"Amplitude"=20.0, "Phase Shift"=0.25, "Zero Position"=0.0}, {"Amplitude"=20.0, "Phase Shift"=0.25, "Zero Position"=0.0}, {"Amplitude"=20.0, "Phase Shift"=0.25, "Zero Position"=0.0}, {"Amplitude"=20.0, "Phase Shift"=0.25, "Zero Position"=0.0}, {"Amplitude"=20.0, "Phase Shift"=0.25, "Zero Position"=0.0}], "Frequency\n& Direction"=0.7, "General A, PS, ZP"={"Amplitude"=20.0, "Phase Shift"=0.25, "Zero Position"=0.0}}] ("Individual Steering")) -> (error out=w34:errorcluster)  [unwired: 1 in, 1 out]
      n16 = property on="IndividualSteering_f(x)" class="Enum (strict)"(error in=w34, "Val(Sgnl)"=IndividualSteering_f(x)_enum."sin(x)" ("Value (Signaling)")) -> (error out=w39:errorcluster)  [unwired: 1 in, 1 out]
      n17 = property on="Fin Status" class="Arr (strict)"(error in=w39, "Value"=T1 [16777215, 16777215, 16777215, 16777215] ("Fin Status")) -> (error out=w90:errorcluster)  [unwired: 1 in, 1 out]
      n18 = property on="SpaceMouse_EnableInputs" class="Clust (strict)"(error in=w90, "Val(Sgnl)"=T23 {"X"=TRUE, "Y"=TRUE, "Z"=TRUE, "phi"=TRUE, "theta"=TRUE, "psi"=TRUE, "All Inputs"=TRUE} ("SpaceMouse_EnableInputs")) -> (error out=w31:errorcluster)  [unwired: 1 in, 1 out]
      n19 = property on="Individual Steering Configurations" class="Clust (strict)"(error in=w31, "Value"=T10 {"Standard"=FALSE, "Left Curve"=FALSE, "Screw"=FALSE, "Inclined"=FALSE, "Looping"=FALSE, "Cuttle"=FALSE} ("Individual Steering Configurations")) -> (error out=w30:errorcluster)  [unwired: 1 in, 1 out]
      n20 = property on="Camera" class="Bool (strict)"(error in=w30, "Val(Sgnl)"=TRUE ("Value (Signaling)")) -> (error out=w47:errorcluster)  [unwired: 1 in, 1 out]
      n21 = property on="Laser" class="Bool (strict)"(error in=w47, "Val(Sgnl)"=FALSE ("Value (Signaling)")) -> (error out=w46:errorcluster)  [unwired: 1 in, 1 out]
      n22 = property on="STOP_LiveStream" class="Bool (strict)"(error in=w46, "Value"=TRUE ("STOP_LiveStream")) -> (error out=w58:errorcluster)  [unwired: 1 in, 1 out]
      n23 = property on="Record Button" class="Bool (strict)"(error in=w58, "Value"=w16) -> (error out=w57:errorcluster)  [unwired: 1 in, 1 out]
      n24 = property on="Picture Button" class="Bool (strict)"(error in=w57, "Value"=w16) -> (error out=w56:errorcluster)  [unwired: 1 in, 1 out]
      n25 = property on="Collision\nDetection" class="Bool (strict)"(error in=w56, "Value"=w16) -> (error out=w21:errorcluster)  [unwired: 1 in, 1 out]
      n26 = property on="Collision\nAvoidance" class="Bool (strict)"(error in=w21, "Value"=w16) -> (error out=w20:errorcluster)  [unwired: 1 in, 1 out]
      n27 = property on="Overlay" class="Bool (strict)"(error in=w20, "Value"=w16) -> (error out=w55:errorcluster)  [unwired: 1 in, 1 out]
      n28 = property on="Collision" class="Bool (strict)"(error in=w55, "Value"=w16) -> (error out=w19:errorcluster)  [unwired: 1 in, 1 out]
      n29 = property on="Laser Detected" class="Bool (strict)"(error in=w19, "Value"=w16) -> (error out=w18:errorcluster)  [unwired: 1 in, 1 out]
      n30 = call "Attitude Control Open.vi"("Scene Graph"=w68) -> ("Attitude Control Handle"=w69:T35)  [unwired: 9 in, 1 out]
      n31 = property on="Avoidance" class="Bool (strict)"(error in=w18, "Value"=w16) -> (error out=w17:errorcluster)  [unwired: 1 in, 1 out]
      n32 = property on="STOP_Swimbladder" class="Bool (strict)"(error in=w17, "Value"=TRUE ("STOP_Swimbladder")) -> (error out=w95:errorcluster)  [unwired: 1 in, 1 out]
      n33 = property on="Save Parameters to File" class="Bool (strict)"(error in=w95, "Value"=FALSE ("Save Parameters to File")) -> (error out=w84:errorcluster)  [unwired: 1 in, 1 out]
      n34 = property on="STOP_Steering" class="Bool (strict)"(error in=w84, "Value"=FALSE ("STOP_Steering")) -> (error out=w83:errorcluster)  [unwired: 1 in, 1 out]
      n35 = property on="Load Parameters from File" class="Bool (strict)"(error in=w83, "Value"=FALSE ("Load Parameters from File")) -> (error out=w94:errorcluster)  [unwired: 1 in, 1 out]
      n36 = property on="Max Depth" class="DigNum (strict)"(error in=w94, "Val(Sgnl)"=2.9 ("Max Depth")) -> (error out=w93:errorcluster)  [unwired: 1 in, 1 out]
      n37 = property on="Depth Desired [m]" class="DigNum (strict)"(error in=w93, "Val(Sgnl)"=0.0 ("Depth Desired [m]")) -> (error out=w92:errorcluster)  [unwired: 1 in, 1 out]
      n38 = property on="Sensors State" class="Clust (strict)"(error in=w92, "Val(Sgnl)"=T28 {"Leakage-Sensor_enabled"=TRUE, "IMU_enabled"=TRUE, "Swimbladder Fill-State-Sensor_enabled"=TRUE, "Flow-Sensor_enabled"=FALSE, "Depth-Sensor_enabled"=TRUE, "Current-Sensor_enabled"=TRUE, "Calibrate Depth"=FALSE, "SB_Piston_Stuck_Detect_enabled"=FALSE, "Check_too_Deep_enabled"=FALSE} ("Sensors State")) -> (error out=w88:errorcluster)  [unwired: 1 in, 1 out]
      n39 = property on="Swimbladder Tuning Parameters" class="Clust (strict)"(error in=w88, "Val(Sgnl)"=T11 {"Excessive_Depth_Deviation_Trigger"=0.4, "Neutral Buoancy_x"=0.2, "Ti_Depth_Control"=1e-05, "kp_Depth_Control"=0.3, "Integrator enabled range Depth"=0.15, "Integrator_enable_Range_Motor"=0.03, "kp_Motor"=150.0, "Ti_Motor"=1.72e-05} ("Swimbladder Tuning Parameters")) -> (error out=w80:errorcluster)  [unwired: 1 in, 1 out]
      n40 = shared-variable "myRIO\\Library_SpaceMouse.lvlib\\SpaceMouse_Buttons"(T26 {"Idle"=TRUE, "Button Right"=FALSE, "Button Left"=FALSE} ("SpaceMouse_Buttons"), error in=w80) -> (error out=w79:errorcluster)
      n41 = property on="SpaceMouse_Parameters" class="Clust (strict)"(error in=w79, "Val(Sgnl)"=T27 {"Lowpass Filter Cutoff Frequency"=10.0, "Idle Threshold"=50.0, "Deadzone"=15000.0, "Filter Sample Size"=25, "FilterOff"=FALSE, "IntegratorOff"=FALSE} ("Value (Signaling)")) -> (error out=w82:errorcluster)  [unwired: 1 in, 1 out]
      n42 = property on="Sepios General Parameters" class="Clust (strict)"(error in=w82, "Val(Sgnl)"=T31 {"Sensors-Settings"={"Water density [kg/m3]"=1000.0, "SB_parameters"={"x0"=0.0, "U_full"=0.695, "U_empty"=3.67}}, "Startup"={"Enable Swimbladder"=FALSE}, "Default Configuration File"=path ""} ("Value (Signaling)")) -> (error out=w77:errorcluster)  [unwired: 1 in, 1 out]
      n43 = property on="SpaceMouse_Refresh" class="Bool (strict)"(error in=w77, "Value"=FALSE ("SpaceMouse_Refresh")) -> (error out=w22:errorcluster)  [unwired: 1 in, 1 out]
      n44 = property on="Velocity Controllers Parameters" class="Clust (strict)"(error in=w22, "Val(Sgnl)"=T15 {"ARW on"={"Phi"=TRUE, "Theta"=TRUE, "Psi"=TRUE}, "kp"={"kp Phi"=0.0, "kp Theta"=0.0, "kp Psi"=0.0}, "Ti"={"Ti Phi"=0.0, "Ti Theta"=0.0, "Ti Psi"=0.0}, "Integrator enabled range [rad      "={"I_E Phi"=0.0, "I_E Theta"=0.0, "I_E Psi"=0.0}} ("Value (Signaling)")) -> (error out=w23:errorcluster)  [unwired: 1 in, 1 out]
      n45 = property on="Velocity Control on" class="Bool (strict)"(error in=w23, "Val(Sgnl)"=FALSE ("Value (Signaling)")) -> (error out=w27:errorcluster)  [unwired: 1 in, 1 out]
      n46 = property on="Flow_LED" class="Bool (strict)"(error in=w27, "Val(Sgnl)"=FALSE ("Value (Signaling)")) -> (error out=w26:errorcluster)  [unwired: 1 in, 1 out]
      n47 = property on="Attitude Control On" class="Bool (strict)"(error in=w26, "Val(Sgnl)"=FALSE ("Value (Signaling)")) -> (error out=w65:errorcluster)  [unwired: 1 in, 1 out]
      n48 = property on="Auto stable when idle" class="Bool (strict)"(error in=w65, "Value"=FALSE ("Auto stable when idle")) -> (error out=w63:errorcluster)  [unwired: 1 in, 1 out]
      n49 = property on="Attitude_Increase_Speed [rad]" class="DigNum (strict)"(error in=w63, "Value"=0.01 ("Attitude_Increase_Speed")) -> (error out=w62:errorcluster)  [unwired: 1 in, 1 out]
      n50 = property on="Attitude Controllers Parameters" class="Clust (strict)"(error in=w62, "Val(Sgnl)"=T15 {"ARW on"={"Phi"=TRUE, "Theta"=TRUE, "Psi"=TRUE}, "kp"={"kp Phi"=4.0, "kp Theta"=8.0, "kp Psi"=5.0}, "Ti"={"Ti Phi"=0.2, "Ti Theta"=0.01, "Ti Psi"=0.01}, "Integrator enabled range [rad      "={"I_E Phi"=0.4, "I_E Theta"=0.2, "I_E Psi"=0.2}} ("Value (Signaling)")) -> (error out=w52:errorcluster)  [unwired: 1 in, 1 out]
      n51 = property on="Intuitive Steering Attitude Control" class="Clust (strict)"(error in=w52, "Val(Sgnl)"=T7 {"Frequency (Hz):"=0.8, "Max. Amplitude (°):"=40.0, "Phase Shift (/Pi):"=0.25, "Flap (°):"=20.0, "Flap Saturation:"=0.7} ("Value (Signaling)")) -> (error out=w53:errorcluster)  [unwired: 1 in, 1 out]
      n52 = property on="EKF_Settings" class="Clust (strict)"(error in=w53, "Val(Sgnl)"=T13 {"Gravity constant"=-9.808205458883663, "Filter Version"=enum."IMU, Pressure, Compass", "Initial Biases"={"Gyro_Bias_nit_x"=0.00198, "Gyro_Bias_init_y"=0.0053, "Gyro_Bias_init_z"=0.0009, "Acc_Bias_init_x"=0.0, "Acc_Bias_init_y"=0.0, "Acc_Bias_init_z"=0.0}, "Use Compass on initialisation"=TRUE, "Initial Biases Covariances"={"Initial_covariance_Gyro_Bias"=0.0014, "Initial_covariance_Acc_Bias"=0.2}, "Magnetic-Field-Vector [utesla]"={"Magf_N_x"=21.565, "Magf_N_y"=0.6833, "Magf_N_z"=42.6149}, "IMU_Sigmas"={"Sigma_w"=0.00033937, "Sigma_wb"=3.8785e-05, "Sigma_a"=0.02, "Sigma_ab"=0.03, "Sigma_m"=1000.0}, "Measurement Sigmas"={"Sigma_v"=500.0, "Sigma_depth"=0.2}} ("Value (Signaling)")) -> (error out=w51:errorcluster)  [unwired: 1 in, 1 out]
      n53 = call "Attitude Control Open.vi"("Scene Graph"=w76) -> ("Attitude Control Handle"=w75:T35)  [unwired: 9 in, 1 out]
    }
    frame #2 {
      # "Wait Startup"
      n54 = Wait (ms)(milliseconds to wait=u32 50) -> ()  [unwired: 1 out]
    }
    frame #3 {
      # "Run"
      n55 = while {
        shift-right: [w277] -> _
        shift-left: TRUE ("All Inputs") -> [w276]
        shift-right: [w259] -> w120
        shift-left: w118 -> [w260]
        tunnel: w114 -> [w266]
        shift-right: [w257] -> _
        shift-left: T33 {"New attitude phi"=0.0, "New attitude theta"=0.0, "New attitude psi"=0.0} ("New desired Attitude") -> [w256]
        stop <- w271 stop-if-true
        # "sehr aufwändig gemacht, for loop wenn Änderung?"
        # "Space Mouse Manager"
        n56 = shared-variable "myRIO\\Library_Steering.lvlib\\Library_AttitudeControl.lvlib\\Attitude Control On"(error in=w266) -> (w269:bool, error out=w265:errorcluster)
        n57 = shared-variable "myRIO\\Library_SpaceMouse.lvlib\\SpaceMouse_FilteredInput"(error in=w265) -> (w268:T36, error out=w254:errorcluster)
        n58 = shared-variable "myRIO\\Library_SpaceMouse.lvlib\\SpaceMouse_Buttons"(error in=w254) -> (w251:T26, error out=w249:errorcluster)
        "SpaceMouse_Buttons" <- w251
        n59 = Unbundle By Name(w251) -> ("Idle"=w250:bool)
        n60 = case shown="False" "Auto stable when idle" {
          tunnel: w250 -> [_ w308]
          tunnel: w249 -> [w305 w307]
          tunnel: [w305 w306] -> w248
          frame False {
          }
          frame True {
            n61 = property on="Attitude Control On" class="Bool (strict)"(error in=w307, "Val(Sgnl)"=w308) -> (error out=w306:errorcluster)  [unwired: 1 in, 1 out]
          }
        }
        n62 = case shown="True" w250 {
          tunnel: w248 -> [w312 w313]
          tunnel: [w310 w313] -> w253
          frame False {
            n63 = shared-variable "myRIO\\Library_Swimbladder.lvlib\\Depth Desired"(error in=w312) -> (w309:dbl, error out=w311:errorcluster)
            n64 = property on="Depth Desired [m]" class="DigNum (strict)"(error in=w311, "Value"=w309) -> (error out=w310:errorcluster)  [unwired: 1 in, 1 out]
          }
          frame True {
          }
        }
        n65 = call "Handle_Space_Mouse_Input.vi"("SpaceMouse_Buttons"=w251, "SpaceMouse_FilteredInput in"=w268, "error in (no error)"=w253, "Attitude_Increase_Speed"="Attitude_Increase_Speed [rad]", "old desired Attitude"=w256, "Attitude Control on"=w269) -> ("error out"=w258:errorcluster, "New desired Attitude"=w257:T33, "SpaceMouse or Controller Output"=w267:T36)  [unwired: 3 in]
        "Filtered Input" <- w267
        n66 = call "Attitude Control Write.vi"("error in (no error)"=w258, "Attitude in radians"=w257, "Attitude Control Handle In"=w260) -> ("error out"=w261:errorcluster, "Attitude Control Handle Out"=w259:T35)  [unwired: 7 in]
        n67 = shared-variable "myRIO\\Library_SpaceMouse.lvlib\\SpaceMouse_RawInput"(error in=w261) -> (→"Raw Input":T37, error out=w252:errorcluster)
        n68 = property on="User Steering Inputs" class="Clust (strict)"(error in=w252) -> (error out=w264:errorcluster, "Value"=w304:T32)  [unwired: 1 in, 1 out]
        n69 = Unbundle(w267) -> ("X"=w280:dbl, "Y"=w283:dbl, "Z"=w286:dbl, "phi"=w289:dbl, "theta"=w292:dbl, "psi"=w295:dbl)
        n70 = Unbundle(w304) -> ("X"=w281:dbl, "Y"=w284:dbl, "Z"=w287:dbl, "phi"=w290:dbl, "theta"=w293:dbl, "psi"=w296:dbl)
        n71 = Unbundle("SpaceMouse_EnableInputs") -> ("X"=w279:bool, "Y"=w282:bool, "Z"=w285:bool, "phi"=w288:bool, "theta"=w291:bool, "psi"=w294:bool, "All Inputs"=w277:bool)
        n72 = Select(t=w280, s=w279, f=w281) -> (s? t:f=w298:dbl)
        n73 = Select(t=w283, s=w282, f=w284) -> (s? t:f=w299:dbl)
        n74 = Select(t=w286, s=w285, f=w287) -> (s? t:f=w300:dbl)
        n75 = Select(t=w289, s=w288, f=w290) -> (s? t:f=w301:dbl)
        n76 = Select(t=w292, s=w291, f=w293) -> (s? t:f=w302:dbl)
        n77 = Select(t=w295, s=w294, f=w296) -> (s? t:f=w303:dbl)
        n78 = Equal?(x=w277, y=w276) -> (x = y?=w275:bool)
        n79 = Bundle("All Inputs"=w277, "All Inputs"=w277, "All Inputs"=w277, "All Inputs"=w277, "All Inputs"=w277, "All Inputs"=w277, "All Inputs"=w277) -> (w274:T38)  [unwired: 1 in]
        n80 = Bundle("X"=w298, "Y"=w299, "Z"=w300, "phi"=w301, "theta"=w302, "psi"=w303) -> (w297:T25)  [unwired: 1 in]
        n81 = Select(t="SpaceMouse_EnableInputs", s=w275, f=w274) -> (s? t:f=w273:T38)
        n82 = property on="User Steering Inputs" class="Clust (strict)"(error in=w264, "Value"=w297) -> (error out=w263:errorcluster)  [unwired: 1 in, 1 out]
        n83 = property on="SpaceMouse_EnableInputs" class="Clust (strict)"(error in=w263, "Value"=w273) -> (error out=w262:errorcluster)  [unwired: 1 in, 1 out]
        n84 = shared-variable "myRIO\\Library_General.lvlib\\Exit"(error in=w262) -> (w271:bool)  [unwired: 1 out]
        n85 = Wait (ms)(milliseconds to wait=u32 50) -> ()  [unwired: 1 out]
      }
      n86 = while {
        tunnel: [w426] -> w128
        tunnel: w114 -> [w424]
        stop <- w429 stop-if-true
        # "Monitor Controls @ 100 Hz"
        n87 = shared-variable "myRIO\\Library_Steering.lvlib\\User Steering Inputs"("User Steering Inputs", error in=w424) -> (error out=w422:errorcluster)
        n88 = case shown="\"Individually\"" "Steering Mode" {
          tunnel: w422 -> [w430 w431 w433]
          tunnel: [w430 w431 w432] -> w421
          frame "Intuitive Steering", Default {
          }
          frame "Control Allocation" {
          }
          frame "Individually" {
            # "to improve..."
            n89 = shared-variable "myRIO\\Library_Steering.lvlib\\Individual Steering"("Individual Steering", error in=w433) -> (error out=w432:errorcluster)
          }
        }
        n90 = event shown="[1] \"Standby\": Value Change" {
          selector: _ -> [_ _ _ _ _ _ _ _ _ _ _ _ _ _ _ _ _ _ _ _ _ _ _ _ _ _ _ _ _ _ _ _ _ _ _]
          dyn-events: _ -> [_ _ _ _ _ _ _ _ _ _ _ _ _ _ _ _ _ _ _ _ _ _ _ _ _ _ _ _ _ _ _ _ _ _ _]
          timeout: 10 -> [_ _ _ _ _ _ _ _ _ _ _ _ _ _ _ _ _ _ _ _ _ _ _ _ _ _ _ _ _ _ _ _ _ _ _]
          tunnel: [w435 w446 w476 w484 w493 w502 w511 w520 w529 w535 w541 w546 w560 w573 w578 w585 w594 w604 w623 w639 w642 w645 w649 w652 w654 w657 w659 w663 w665 w668 w672 w675 w678 w682 w685] -> w428
          tunnel: w421 -> [w435 w445 w475 w485 w495 w504 w513 w521 w530 w536 w543 w545 w562 w572 w579 w589 w595 w599 w618 w637 w641 w644 w648 w651 w655 w656 w660 w664 w666 w669 w671 w674 w677 w681 w684]
          event Timeout {
            n91 = event-data() -> ()  [unwired: 1 in, 3 out]
          }
          event "Standby": Value Change {
            n92 = event-data() -> ("NewVal"=w438:bool)  [unwired: 1 in, 5 out]
            n93 = case shown="False" w438 {
              selector: w438 -> [_ w470]
              tunnel: [w469 w470] -> w449
              tunnel: [w468 w470] -> w448
              tunnel: [w467 w470] -> w447
              tunnel: w445 -> [w464 w472]
              tunnel: [w460 w474] -> w444
              tunnel: [w463 w470] -> w439
              frame False {
                n94 = property on="STOP_Steering" class="Bool (strict)"(error in=w464) -> (error out=w466:errorcluster, "Value"=w469:bool)  [unwired: 1 in, 1 out]
                n95 = property on="STOP_Swimbladder" class="Bool (strict)"(error in=w466) -> (error out=w465:errorcluster, "Value"=w468:bool)  [unwired: 1 in, 1 out]
                n96 = property on="STOP_LiveStream" class="Bool (strict)"(error in=w465) -> (error out=w461:errorcluster, "Value"=w467:bool)  [unwired: 1 in, 1 out]
                n97 = property on="Collision\nAvoidance" class="Bool (strict)"(error in=w461) -> (error out=w460:errorcluster, "Value"=w462:bool)  [unwired: 1 in, 1 out]
                n98 = Not(x=w462) -> (.not. x?=w463:bool)
              }
              frame True {
                w473 = FALSE ("Reached Standby")
                n99 = property on="Standby" class="Bool (strict)"(error in=w472, "Visible"=w473) -> (error out=w471:errorcluster)  [unwired: 1 in, 1 out]
                n100 = shared-variable "myRIO\\Library_General.lvlib\\Reached Standby"(w473, error in=w471) -> (error out=w474:errorcluster)
              }
            }
            n101 = shared-variable "myRIO\\Library_General.lvlib\\Standby"(w438, error in=w444) -> (error out=w437:errorcluster)
            n102 = shared-variable "myRIO\\Library_Log.lvlib\\STOP_Log"(w438, error in=w437) -> (error out=w436:errorcluster)
            n103 = shared-variable "myRIO\\Library_Steering.lvlib\\STOP_Steering"(w449, error in=w436) -> (error out=w451:errorcluster)
            n104 = Wait (ms)(milliseconds to wait=u32 1000) -> (millisecond timer value=w442:u32)
            n105 = shared-variable "myRIO\\Library_Swimbladder.lvlib\\STOP_Swimbladder"(w448, error in=w451) -> (error out=w450:errorcluster)
            n106 = shared-variable "myRIO\\Library_Sensors.lvlib\\STOP_LiveStream"(w447, error in=w450) -> (error out=w441:errorcluster)
            n107 = shared-variable "myRIO\\Library_Steering.lvlib\\Library_CollisionDetection.lvlib\\STOP_CollisionAvoidance"(w439, error in=w441) -> (error out=w440:errorcluster)
            n108 = case shown="True" w438 {
              tunnel: w440 -> [w452 w454]
              tunnel: [w452 w455] -> w446
              tunnel: w442 -> [_ _]
              frame False {
              }
              frame True {
                n109 = while {
                  tunnel: w454 -> [w459]
                  tunnel: [w458] -> w455
                  tunnel: [w456] -> w453
                  stop <- w456 stop-if-true
                  n110 = shared-variable "myRIO\\Library_General.lvlib\\Reached Standby"(error in=w459) -> (w456:bool, error out=w458:errorcluster)
                  n111 = Wait (ms)(milliseconds to wait=u32 10) -> ()  [unwired: 1 out]
                }
                n112 = property on="Standby" class="Bool (strict)"("Visible"=w453) -> ()  [unwired: 2 in, 2 out]
              }
            }
          }
          event Value Change {
            n113 = event-data() -> ("NewVal"=w479:bool)  [unwired: 1 in, 5 out]
            n114 = case shown="True" w479 {
              tunnel: [w480 w482] -> w478
              tunnel: w475 -> [w480 w481]
              frame False {
              }
              frame True {
                n115 = property on="Individual Steering" class="Arr (strict)"(error in=w481, "Val(Sgnl)"=T9 [{"Fin Parameters"=[{"Amplitude"=25.0, "Phase Shift"=0.25, "Zero Position"=0.0}, {"Amplitude"=25.0, "Phase Shift"=0.25, "Zero Position"=0.0}, {"Amplitude"=25.0, "Phase Shift"=0.25, "Zero Position"=0.0}, {"Amplitude"=25.0, "Phase Shift"=0.25, "Zero Position"=0.0}, {"Amplitude"=25.0, "Phase Shift"=0.25, "Zero Position"=0.0}, {"Amplitude"=25.0, "Phase Shift"=0.25, "Zero Position"=0.0}, {"Amplitude"=25.0, "Phase Shift"=0.25, "Zero Position"=0.0}, {"Amplitude"=25.0, "Phase Shift"=0.25, "Zero Position"=0.0}, {"Amplitude"=25.0, "Phase Shift"=0.25, "Zero Position"=0.0}], "Frequency\n& Direction"=0.7, "General A, PS, ZP"={"Amplitude"=20.0, "Phase Shift"=0.25, "Zero Position"=0.0}}, {"Fin Parameters"=[{"Amplitude"=25.0, "Phase Shift"=0.25, "Zero Position"=0.0}, {"Amplitude"=25.0, "Phase Shift"=0.25, "Zero Position"=0.0}, {"Amplitude"=25.0, "Phase Shift"=0.25, "Zero Position"=0.0}, {"Amplitude"=25.0, "Phase Shift"=0.25, "Zero Position"=0.0}, {"Amplitude"=25.0, "Phase Shift"=0.25, "Zero Position"=0.0}, {"Amplitude"=25.0, "Phase Shift"=0.25, "Zero Position"=0.0}, {"Amplitude"=25.0, "Phase Shift"=0.25, "Zero Position"=0.0}, {"Amplitude"=25.0, "Phase Shift"=0.25, "Zero Position"=0.0}, {"Amplitude"=25.0, "Phase Shift"=0.25, "Zero Position"=0.0}], "Frequency\n& Direction"=0.7, "General A, PS, ZP"={"Amplitude"=20.0, "Phase Shift"=0.25, "Zero Position"=0.0}}, {"Fin Parameters"=[{"Amplitude"=25.0, "Phase Shift"=0.25, "Zero Position"=0.0}, {"Amplitude"=25.0, "Phase Shift"=0.25, "Zero Position"=0.0}, {"Amplitude"=25.0, "Phase Shift"=0.25, "Zero Position"=0.0}, {"Amplitude"=25.0, "Phase Shift"=0.25, "Zero Position"=0.0}, {"Amplitude"=25.0, "Phase Shift"=0.25, "Zero Position"=0.0}, {"Amplitude"=25.0, "Phase Shift"=0.25, "Zero Position"=0.0}, {"Amplitude"=25.0, "Phase Shift"=0.25, "Zero Position"=0.0}, {"Amplitude"=25.0, "Phase Shift"=0.25, "Zero Position"=0.0}, {"Amplitude"=25.0, "Phase Shift"=0.25, "Zero Position"=0.0}], "Frequency\n& Direction"=0.7, "General A, PS, ZP"={"Amplitude"=20.0, "Phase Shift"=0.25, "Zero Position"=0.0}}, {"Fin Parameters"=[{"Amplitude"=25.0, "Phase Shift"=0.25, "Zero Position"=0.0}, {"Amplitude"=25.0, "Phase Shift"=0.25, "Zero Position"=0.0}, {"Amplitude"=25.0, "Phase Shift"=0.25, "Zero Position"=0.0}, {"Amplitude"=25.0, "Phase Shift"=0.25, "Zero Position"=0.0}, {"Amplitude"=25.0, "Phase Shift"=0.25, "Zero Position"=0.0}, {"Amplitude"=25.0, "Phase Shift"=0.25, "Zero Position"=0.0}, {"Amplitude"=25.0, "Phase Shift"=0.25, "Zero Position"=0.0}, {"Amplitude"=25.0, "Phase Shift"=0.25, "Zero Position"=0.0}, {"Amplitude"=25.0, "Phase Shift"=0.25, "Zero Position"=0.0}], "Frequency\n& Direction"=0.7, "General A, PS, ZP"={"Amplitude"=20.0, "Phase Shift"=0.25, "Zero Position"=0.0}}] ("Value (Signaling)")) -> (error out=w482:errorcluster)  [unwired: 1 in, 1 out]
              }
            }
            n116 = property on="Individual Steering Configurations" class="Clust (strict)"(error in=w478, "Value"=T10 {"Standard"=FALSE, "Left Curve"=FALSE, "Screw"=FALSE, "Inclined"=FALSE, "Looping"=FALSE, "Cuttle"=FALSE} ("Individual Steering Configurations")) -> (error out=w476:errorcluster)  [unwired: 1 in, 1 out]
          }
          event Value Change {
            n117 = event-data() -> ("NewVal"=w486:bool)  [unwired: 1 in, 5 out]
            n118 = case shown="True" w486 {
              tunnel: [w489 w491] -> w488
              tunnel: w485 -> [w489 w490]
              frame False {
              }
              frame True {
                n119 = property on="Individual Steering" class="Arr (strict)"(error in=w490, "Val(Sgnl)"=T9 [{"Fin Parameters"=[{"Amplitude"=30.0, "Phase Shift"=0.25, "Zero Position"=0.0}, {"Amplitude"=30.0, "Phase Shift"=0.25, "Zero Position"=0.0}, {"Amplitude"=30.0, "Phase Shift"=0.25, "Zero Position"=0.0}, {"Amplitude"=30.0, "Phase Shift"=0.25, "Zero Position"=0.0}, {"Amplitude"=30.0, "Phase Shift"=0.25, "Zero Position"=0.0}, {"Amplitude"=30.0, "Phase Shift"=0.25, "Zero Position"=0.0}, {"Amplitude"=30.0, "Phase Shift"=0.25, "Zero Position"=0.0}, {"Amplitude"=30.0, "Phase Shift"=0.25, "Zero Position"=0.0}, {"Amplitude"=30.0, "Phase Shift"=0.25, "Zero Position"=0.0}], "Frequency\n& Direction"=0.9, "General A, PS, ZP"={"Amplitude"=20.0, "Phase Shift"=0.25, "Zero Position"=0.0}}, {"Fin Parameters"=[{"Amplitude"=30.0, "Phase Shift"=0.25, "Zero Position"=0.0}, {"Amplitude"=30.0, "Phase Shift"=0.25, "Zero Position"=0.0}, {"Amplitude"=30.0, "Phase Shift"=0.25, "Zero Position"=0.0}, {"Amplitude"=30.0, "Phase Shift"=0.25, "Zero Position"=0.0}, {"Amplitude"=30.0, "Phase Shift"=0.25, "Zero Position"=0.0}, {"Amplitude"=30.0, "Phase Shift"=0.25, "Zero Position"=0.0}, {"Amplitude"=30.0, "Phase Shift"=0.25, "Zero Position"=0.0}, {"Amplitude"=30.0, "Phase Shift"=0.25, "Zero Position"=0.0}, {"Amplitude"=30.0, "Phase Shift"=0.25, "Zero Position"=0.0}], "Frequency\n& Direction"=0.9, "General A, PS, ZP"={"Amplitude"=20.0, "Phase Shift"=0.25, "Zero Position"=0.0}}, {"Fin Parameters"=[{"Amplitude"=30.0, "Phase Shift"=0.25, "Zero Position"=0.0}, {"Amplitude"=30.0, "Phase Shift"=0.25, "Zero Position"=0.0}, {"Amplitude"=30.0, "Phase Shift"=0.25, "Zero Position"=0.0}, {"Amplitude"=30.0, "Phase Shift"=0.25, "Zero Position"=0.0}, {"Amplitude"=30.0, "Phase Shift"=0.25, "Zero Position"=0.0}, {"Amplitude"=30.0, "Phase Shift"=0.25, "Zero Position"=0.0}, {"Amplitude"=30.0, "Phase Shift"=0.25, "Zero Position"=0.0}, {"Amplitude"=30.0, "Phase Shift"=0.25, "Zero Position"=0.0}, {"Amplitude"=30.0, "Phase Shift"=0.25, "Zero Position"=0.0}], "Frequency\n& Direction"=0.9, "General A, PS, ZP"={"Amplitude"=20.0, "Phase Shift"=0.25, "Zero Position"=0.0}}, {"Fin Parameters"=[{"Amplitude"=30.0, "Phase Shift"=0.25, "Zero Position"=0.0}, {"Amplitude"=30.0, "Phase Shift"=0.25, "Zero Position"=0.0}, {"Amplitude"=30.0, "Phase Shift"=0.25, "Zero Position"=0.0}, {"Amplitude"=30.0, "Phase Shift"=0.25, "Zero Position"=0.0}, {"Amplitude"=30.0, "Phase Shift"=0.25, "Zero Position"=0.0}, {"Amplitude"=30.0, "Phase Shift"=0.25, "Zero Position"=0.0}, {"Amplitude"=30.0, "Phase Shift"=0.25, "Zero Position"=0.0}, {"Amplitude"=30.0, "Phase Shift"=0.25, "Zero Position"=0.0}, {"Amplitude"=30.0, "Phase Shift"=0.25, "Zero Position"=0.0}], "Frequency\n& Direction"=-0.9, "General A, PS, ZP"={"Amplitude"=20.0, "Phase Shift"=0.25, "Zero Position"=0.0}}] ("Value (Signaling)")) -> (error out=w491:errorcluster)  [unwired: 1 in, 1 out]
              }
            }
            n120 = property on="Individual Steering Configurations" class="Clust (strict)"(error in=w488, "Value"=T10 {"Standard"=FALSE, "Left Curve"=FALSE, "Screw"=FALSE, "Inclined"=FALSE, "Looping"=FALSE, "Cuttle"=FALSE} ("Individual Steering Configurations")) -> (error out=w484:errorcluster)  [unwired: 1 in, 1 out]
          }
          event Value Change {
            n121 = event-data() -> ("NewVal"=w494:bool)  [unwired: 1 in, 5 out]
            n122 = case shown="True" w494 {
              tunnel: [w498 w500] -> w497
              tunnel: w495 -> [w498 w499]
              frame False {
              }
              frame True {
                n123 = property on="Individual Steering" class="Arr (strict)"(error in=w499, "Val(Sgnl)"=T9 [{"Fin Parameters"=[{"Amplitude"=0.0, "Phase Shift"=0.0, "Zero Position"=45.0}, {"Amplitude"=0.0, "Phase Shift"=0.0, "Zero Position"=40.0}, {"Amplitude"=0.0, "Phase Shift"=0.0, "Zero Position"=30.0}, {"Amplitude"=0.0, "Phase Shift"=0.0, "Zero Position"=15.0}, {"Amplitude"=0.0, "Phase Shift"=0.0, "Zero Position"=0.0}, {"Amplitude"=0.0, "Phase Shift"=0.0, "Zero Position"=-15.0}, {"Amplitude"=0.0, "Phase Shift"=0.0, "Zero Position"=-30.0}, {"Amplitude"=0.0, "Phase Shift"=0.0, "Zero Position"=-40.0}, {"Amplitude"=0.0, "Phase Shift"=0.0, "Zero Position"=-45.0}], "Frequency\n& Direction"=0.9, "General A, PS, ZP"={"Amplitude"=20.0, "Phase Shift"=0.25, "Zero Position"=0.0}}, {"Fin Parameters"=[{"Amplitude"=30.0, "Phase Shift"=0.25, "Zero Position"=0.0}, {"Amplitude"=30.0, "Phase Shift"=0.25, "Zero Position"=0.0}, {"Amplitude"=30.0, "Phase Shift"=0.25, "Zero Position"=0.0}, {"Amplitude"=30.0, "Phase Shift"=0.25, "Zero Position"=0.0}, {"Amplitude"=30.0, "Phase Shift"=0.25, "Zero Position"=0.0}, {"Amplitude"=30.0, "Phase Shift"=0.25, "Zero Position"=0.0}, {"Amplitude"=30.0, "Phase Shift"=0.25, "Zero Position"=0.0}, {"Amplitude"=30.0, "Phase Shift"=0.25, "Zero Position"=0.0}, {"Amplitude"=30.0, "Phase Shift"=0.25, "Zero Position"=0.0}], "Frequency\n& Direction"=0.9, "General A, PS, ZP"={"Amplitude"=20.0, "Phase Shift"=0.25, "Zero Position"=0.0}}, {"Fin Parameters"=[{"Amplitude"=0.0, "Phase Shift"=0.0, "Zero Position"=45.0}, {"Amplitude"=0.0, "Phase Shift"=0.0, "Zero Position"=40.0}, {"Amplitude"=0.0, "Phase Shift"=0.0, "Zero Position"=30.0}, {"Amplitude"=0.0, "Phase Shift"=0.0, "Zero Position"=15.0}, {"Amplitude"=0.0, "Phase Shift"=0.0, "Zero Position"=0.0}, {"Amplitude"=0.0, "Phase Shift"=0.0, "Zero Position"=-15.0}, {"Amplitude"=0.0, "Phase Shift"=0.0, "Zero Position"=-30.0}, {"Amplitude"=0.0, "Phase Shift"=0.0, "Zero Position"=-40.0}, {"Amplitude"=0.0, "Phase Shift"=0.0, "Zero Position"=-45.0}], "Frequency\n& Direction"=0.9, "General A, PS, ZP"={"Amplitude"=20.0, "Phase Shift"=0.25, "Zero Position"=0.0}}, {"Fin Parameters"=[{"Amplitude"=30.0, "Phase Shift"=0.25, "Zero Position"=0.0}, {"Amplitude"=30.0, "Phase Shift"=0.25, "Zero Position"=0.0}, {"Amplitude"=30.0, "Phase Shift"=0.25, "Zero Position"=0.0}, {"Amplitude"=30.0, "Phase Shift"=0.25, "Zero Position"=0.0}, {"Amplitude"=30.0, "Phase Shift"=0.25, "Zero Position"=0.0}, {"Amplitude"=30.0, "Phase Shift"=0.25, "Zero Position"=0.0}, {"Amplitude"=30.0, "Phase Shift"=0.25, "Zero Position"=0.0}, {"Amplitude"=30.0, "Phase Shift"=0.25, "Zero Position"=0.0}, {"Amplitude"=30.0, "Phase Shift"=0.25, "Zero Position"=0.0}], "Frequency\n& Direction"=0.9, "General A, PS, ZP"={"Amplitude"=20.0, "Phase Shift"=0.25, "Zero Position"=0.0}}] ("Value (Signaling)")) -> (error out=w500:errorcluster)  [unwired: 1 in, 1 out]
              }
            }
            n124 = property on="Individual Steering Configurations" class="Clust (strict)"(error in=w497, "Value"=T10 {"Standard"=FALSE, "Left Curve"=FALSE, "Screw"=FALSE, "Inclined"=FALSE, "Looping"=FALSE, "Cuttle"=FALSE} ("Individual Steering Configurations")) -> (error out=w493:errorcluster)  [unwired: 1 in, 1 out]
          }
          event Value Change {
            n125 = event-data() -> ("NewVal"=w503:bool)  [unwired: 1 in, 5 out]
            n126 = case shown="True" w503 {
              tunnel: [w507 w509] -> w506
              tunnel: w504 -> [w507 w508]
              frame False {
              }
              frame True {
                n127 = property on="Individual Steering" class="Arr (strict)"(error in=w508, "Val(Sgnl)"=T9 [{"Fin Parameters"=[{"Amplitude"=20.0, "Phase Shift"=0.25, "Zero Position"=0.0}, {"Amplitude"=20.0, "Phase Shift"=0.25, "Zero Position"=0.0}, {"Amplitude"=20.0, "Phase Shift"=0.25, "Zero Position"=0.0}, {"Amplitude"=20.0, "Phase Shift"=0.25, "Zero Position"=0.0}, {"Amplitude"=20.0, "Phase Shift"=0.25, "Zero Position"=0.0}, {"Amplitude"=20.0, "Phase Shift"=0.25, "Zero Position"=0.0}, {"Amplitude"=20.0, "Phase Shift"=0.25, "Zero Position"=0.0}, {"Amplitude"=20.0, "Phase Shift"=0.25, "Zero Position"=0.0}, {"Amplitude"=20.0, "Phase Shift"=0.25, "Zero Position"=0.0}], "Frequency\n& Direction"=0.9, "General A, PS, ZP"={"Amplitude"=20.0, "Phase Shift"=0.25, "Zero Position"=0.0}}, {"Fin Parameters"=[{"Amplitude"=20.0, "Phase Shift"=0.25, "Zero Position"=20.0}, {"Amplitude"=20.0, "Phase Shift"=0.25, "Zero Position"=15.0}, {"Amplitude"=20.0, "Phase Shift"=0.25, "Zero Position"=10.0}, {"Amplitude"=20.0, "Phase Shift"=0.25, "Zero Position"=5.0}, {"Amplitude"=20.0, "Phase Shift"=0.25, "Zero Position"=0.0}, {"Amplitude"=20.0, "Phase Shift"=0.25, "Zero Position"=-5.0}, {"Amplitude"=20.0, "Phase Shift"=0.25, "Zero Position"=-10.0}, {"Amplitude"=20.0, "Phase Shift"=0.25, "Zero Position"=-15.0}, {"Amplitude"=20.0, "Phase Shift"=0.25, "Zero Position"=-20.0}], "Frequency\n& Direction"=0.9, "General A, PS, ZP"={"Amplitude"=20.0, "Phase Shift"=0.25, "Zero Position"=0.0}}, {"Fin Parameters"=[{"Amplitude"=20.0, "Phase Shift"=0.25, "Zero Position"=0.0}, {"Amplitude"=20.0, "Phase Shift"=0.25, "Zero Position"=0.0}, {"Amplitude"=20.0, "Phase Shift"=0.25, "Zero Position"=0.0}, {"Amplitude"=20.0, "Phase Shift"=0.25, "Zero Position"=0.0}, {"Amplitude"=20.0, "Phase Shift"=0.25, "Zero Position"=0.0}, {"Amplitude"=20.0, "Phase Shift"=0.25, "Zero Position"=0.0}, {"Amplitude"=20.0, "Phase Shift"=0.25, "Zero Position"=0.0}, {"Amplitude"=20.0, "Phase Shift"=0.25, "Zero Position"=0.0}, {"Amplitude"=20.0, "Phase Shift"=0.25, "Zero Position"=0.0}], "Frequency\n& Direction"=0.9, "General A, PS, ZP"={"Amplitude"=20.0, "Phase Shift"=0.25, "Zero Position"=0.0}}, {"Fin Parameters"=[{"Amplitude"=20.0, "Phase Shift"=0.25, "Zero Position"=-20.0}, {"Amplitude"=20.0, "Phase Shift"=0.25, "Zero Position"=-15.0}, {"Amplitude"=20.0, "Phase Shift"=0.25, "Zero Position"=-10.0}, {"Amplitude"=20.0, "Phase Shift"=0.25, "Zero Position"=-5.0}, {"Amplitude"=20.0, "Phase Shift"=0.25, "Zero Position"=0.0}, {"Amplitude"=20.0, "Phase Shift"=0.25, "Zero Position"=5.0}, {"Amplitude"=20.0, "Phase Shift"=0.25, "Zero Position"=10.0}, {"Amplitude"=20.0, "Phase Shift"=0.25, "Zero Position"=15.0}, {"Amplitude"=20.0, "Phase Shift"=0.25, "Zero Position"=20.0}], "Frequency\n& Direction"=0.9, "General A, PS, ZP"={"Amplitude"=20.0, "Phase Shift"=0.25, "Zero Position"=0.0}}] ("Value (Signaling)")) -> (error out=w509:errorcluster)  [unwired: 1 in, 1 out]
              }
            }
            n128 = property on="Individual Steering Configurations" class="Clust (strict)"(error in=w506, "Value"=T10 {"Standard"=FALSE, "Left Curve"=FALSE, "Screw"=FALSE, "Inclined"=FALSE, "Looping"=FALSE, "Cuttle"=FALSE} ("Individual Steering Configurations")) -> (error out=w502:errorcluster)  [unwired: 1 in, 1 out]
          }
          event Value Change {
            n129 = event-data() -> ("NewVal"=w512:bool)  [unwired: 1 in, 5 out]
            n130 = case shown="True" w512 {
              tunnel: [w516 w518] -> w515
              tunnel: w513 -> [w516 w517]
              frame False {
              }
              frame True {
                n131 = property on="Individual Steering" class="Arr (strict)"(error in=w517, "Val(Sgnl)"=T9 [{"Fin Parameters"=[{"Amplitude"=30.0, "Phase Shift"=0.25, "Zero Position"=0.0}, {"Amplitude"=30.0, "Phase Shift"=0.25, "Zero Position"=0.0}, {"Amplitude"=30.0, "Phase Shift"=0.25, "Zero Position"=0.0}, {"Amplitude"=30.0, "Phase Shift"=0.25, "Zero Position"=0.0}, {"Amplitude"=30.0, "Phase Shift"=0.25, "Zero Position"=0.0}, {"Amplitude"=30.0, "Phase Shift"=0.25, "Zero Position"=0.0}, {"Amplitude"=30.0, "Phase Shift"=0.25, "Zero Position"=0.0}, {"Amplitude"=30.0, "Phase Shift"=0.25, "Zero Position"=0.0}, {"Amplitude"=30.0, "Phase Shift"=0.25, "Zero Position"=0.0}], "Frequency\n& Direction"=-0.9, "General A, PS, ZP"={"Amplitude"=20.0, "Phase Shift"=0.25, "Zero Position"=0.0}}, {"Fin Parameters"=[{"Amplitude"=30.0, "Phase Shift"=0.25, "Zero Position"=0.0}, {"Amplitude"=30.0, "Phase Shift"=0.25, "Zero Position"=0.0}, {"Amplitude"=30.0, "Phase Shift"=0.25, "Zero Position"=0.0}, {"Amplitude"=30.0, "Phase Shift"=0.25, "Zero Position"=0.0}, {"Amplitude"=30.0, "Phase Shift"=0.25, "Zero Position"=0.0}, {"Amplitude"=30.0, "Phase Shift"=0.25, "Zero Position"=0.0}, {"Amplitude"=30.0, "Phase Shift"=0.25, "Zero Position"=0.0}, {"Amplitude"=30.0, "Phase Shift"=0.25, "Zero Position"=0.0}, {"Amplitude"=30.0, "Phase Shift"=0.25, "Zero Position"=0.0}], "Frequency\n& Direction"=0.9, "General A, PS, ZP"={"Amplitude"=20.0, "Phase Shift"=0.25, "Zero Position"=0.0}}, {"Fin Parameters"=[{"Amplitude"=30.0, "Phase Shift"=0.25, "Zero Position"=0.0}, {"Amplitude"=30.0, "Phase Shift"=0.25, "Zero Position"=0.0}, {"Amplitude"=30.0, "Phase Shift"=0.25, "Zero Position"=0.0}, {"Amplitude"=30.0, "Phase Shift"=0.25, "Zero Position"=0.0}, {"Amplitude"=30.0, "Phase Shift"=0.25, "Zero Position"=0.0}, {"Amplitude"=30.0, "Phase Shift"=0.25, "Zero Position"=0.0}, {"Amplitude"=30.0, "Phase Shift"=0.25, "Zero Position"=0.0}, {"Amplitude"=30.0, "Phase Shift"=0.25, "Zero Position"=0.0}, {"Amplitude"=30.0, "Phase Shift"=0.25, "Zero Position"=0.0}], "Frequency\n& Direction"=0.9, "General A, PS, ZP"={"Amplitude"=20.0, "Phase Shift"=0.25, "Zero Position"=0.0}}, {"Fin Parameters"=[{"Amplitude"=30.0, "Phase Shift"=0.25, "Zero Position"=0.0}, {"Amplitude"=30.0, "Phase Shift"=0.25, "Zero Position"=0.0}, {"Amplitude"=30.0, "Phase Shift"=0.25, "Zero Position"=0.0}, {"Amplitude"=30.0, "Phase Shift"=0.25, "Zero Position"=0.0}, {"Amplitude"=30.0, "Phase Shift"=0.25, "Zero Position"=0.0}, {"Amplitude"=30.0, "Phase Shift"=0.25, "Zero Position"=0.0}, {"Amplitude"=30.0, "Phase Shift"=0.25, "Zero Position"=0.0}, {"Amplitude"=30.0, "Phase Shift"=0.25, "Zero Position"=0.0}, {"Amplitude"=30.0, "Phase Shift"=0.25, "Zero Position"=0.0}], "Frequency\n& Direction"=0.9, "General A, PS, ZP"={"Amplitude"=20.0, "Phase Shift"=0.25, "Zero Position"=0.0}}] ("Value (Signaling)")) -> (error out=w518:errorcluster)  [unwired: 1 in, 1 out]
              }
            }
            n132 = property on="Individual Steering Configurations" class="Clust (strict)"(error in=w515, "Value"=T10 {"Standard"=FALSE, "Left Curve"=FALSE, "Screw"=FALSE, "Inclined"=FALSE, "Looping"=FALSE, "Cuttle"=FALSE} ("Individual Steering Configurations")) -> (error out=w511:errorcluster)  [unwired: 1 in, 1 out]
          }
          event Value Change {
            n133 = event-data() -> ("NewVal"=w522:bool)  [unwired: 1 in, 5 out]
            n134 = case shown="True" w522 {
              tunnel: [w525 w527] -> w524
              tunnel: w521 -> [w525 w526]
              frame False {
              }
              frame True {
                n135 = property on="Individual Steering" class="Arr (strict)"(error in=w526, "Val(Sgnl)"=T9 [{"Fin Parameters"=[{"Amplitude"=28.0, "Phase Shift"=0.25, "Zero Position"=0.0}, {"Amplitude"=28.0, "Phase Shift"=0.25, "Zero Position"=0.0}, {"Amplitude"=28.0, "Phase Shift"=0.25, "Zero Position"=0.0}, {"Amplitude"=28.0, "Phase Shift"=0.25, "Zero Position"=0.0}, {"Amplitude"=28.0, "Phase Shift"=0.25, "Zero Position"=0.0}, {"Amplitude"=28.0, "Phase Shift"=0.25, "Zero Position"=0.0}, {"Amplitude"=28.0, "Phase Shift"=0.25, "Zero Position"=0.0}, {"Amplitude"=28.0, "Phase Shift"=0.25, "Zero Position"=0.0}, {"Amplitude"=28.0, "Phase Shift"=0.25, "Zero Position"=0.0}], "Frequency\n& Direction"=0.9, "General A, PS, ZP"={"Amplitude"=20.0, "Phase Shift"=0.25, "Zero Position"=0.0}}, {"Fin Parameters"=[{"Amplitude"=28.0, "Phase Shift"=0.25, "Zero Position"=0.0}, {"Amplitude"=28.0, "Phase Shift"=0.25, "Zero Position"=0.0}, {"Amplitude"=28.0, "Phase Shift"=0.25, "Zero Position"=0.0}, {"Amplitude"=28.0, "Phase Shift"=0.25, "Zero Position"=0.0}, {"Amplitude"=28.0, "Phase Shift"=0.25, "Zero Position"=0.0}, {"Amplitude"=28.0, "Phase Shift"=0.25, "Zero Position"=0.0}, {"Amplitude"=28.0, "Phase Shift"=0.25, "Zero Position"=0.0}, {"Amplitude"=28.0, "Phase Shift"=0.25, "Zero Position"=0.0}, {"Amplitude"=28.0, "Phase Shift"=0.25, "Zero Position"=0.0}], "Frequency\n& Direction"=0.9, "General A, PS, ZP"={"Amplitude"=20.0, "Phase Shift"=0.25, "Zero Position"=0.0}}, {"Fin Parameters"=[{"Amplitude"=28.0, "Phase Shift"=0.25, "Zero Position"=0.0}, {"Amplitude"=28.0, "Phase Shift"=0.25, "Zero Position"=0.0}, {"Amplitude"=28.0, "Phase Shift"=0.25, "Zero Position"=0.0}, {"Amplitude"=28.0, "Phase Shift"=0.25, "Zero Position"=0.0}, {"Amplitude"=28.0, "Phase Shift"=0.25, "Zero Position"=0.0}, {"Amplitude"=28.0, "Phase Shift"=0.25, "Zero Position"=0.0}, {"Amplitude"=28.0, "Phase Shift"=0.25, "Zero Position"=0.0}, {"Amplitude"=28.0, "Phase Shift"=0.25, "Zero Position"=0.0}, {"Amplitude"=28.0, "Phase Shift"=0.25, "Zero Position"=0.0}], "Frequency\n& Direction"=0.9, "General A, PS, ZP"={"Amplitude"=20.0, "Phase Shift"=0.25, "Zero Position"=0.0}}, {"Fin Parameters"=[{"Amplitude"=28.0, "Phase Shift"=0.25, "Zero Position"=0.0}, {"Amplitude"=28.0, "Phase Shift"=0.25, "Zero Position"=0.0}, {"Amplitude"=28.0, "Phase Shift"=0.25, "Zero Position"=0.0}, {"Amplitude"=28.0, "Phase Shift"=0.25, "Zero Position"=0.0}, {"Amplitude"=28.0, "Phase Shift"=0.25, "Zero Position"=0.0}, {"Amplitude"=28.0, "Phase Shift"=0.25, "Zero Position"=0.0}, {"Amplitude"=28.0, "Phase Shift"=0.25, "Zero Position"=0.0}, {"Amplitude"=28.0, "Phase Shift"=0.25, "Zero Position"=0.0}, {"Amplitude"=28.0, "Phase Shift"=0.25, "Zero Position"=0.0}], "Frequency\n& Direction"=0.9, "General A, PS, ZP"={"Amplitude"=20.0, "Phase Shift"=0.25, "Zero Position"=0.0}}] ("Value (Signaling)")) -> (error out=w527:errorcluster)  [unwired: 1 in, 1 out]
              }
            }
            n136 = property on="Individual Steering Configurations" class="Clust (strict)"(error in=w524, "Value"=T10 {"Standard"=FALSE, "Left Curve"=FALSE, "Screw"=FALSE, "Inclined"=FALSE, "Looping"=FALSE, "Cuttle"=FALSE} ("Individual Steering Configurations")) -> (error out=w520:errorcluster)  [unwired: 1 in, 1 out]
          }
          event "Create New Log": Value Change {
            n137 = event-data() -> ("NewVal"=w531:bool)  [unwired: 1 in, 5 out]
            n138 = shared-variable "myRIO\\Library_Log.lvlib\\STOP_Log"(w531, error in=w530) -> (error out=w529:errorcluster)
          }
          event "Attitude Control On": Value Change {
            n139 = event-data() -> ("OldVal"=w534:bool, "NewVal"=w533:bool)  [unwired: 1 in, 4 out]
            n140 = Not Equal?(x=w534, y=w533) -> (x != y?=w532:bool)
            n141 = case shown="True" w532 {
              tunnel: w533 -> [_ w540]
              tunnel: w536 -> [w537 w539]
              tunnel: [w537 w538] -> w535
              frame False {
              }
              frame True {
                # "due to signaling when spacemouse in idle and auto-stable on"
                n142 = shared-variable "myRIO\\Library_Steering.lvlib\\Library_AttitudeControl.lvlib\\Attitude Control On"(w540, error in=w539) -> (error out=w538:errorcluster)
              }
            }
          }
          event Value Change {
            n143 = event-data() -> ("NewVal"=w542:T13)  [unwired: 1 in, 5 out]
            n144 = shared-variable "myRIO\\Library_Steering.lvlib\\Library_AttitudeControl.lvlib\\EKF_Settings"(w542, error in=w543) -> (error out=w541:errorcluster)
          }
          event Panel Close {
            w544 = TRUE ("Standby")
            n145 = event-data() -> ()  [unwired: 1 in, 4 out]
            n146 = shared-variable "myRIO\\Library_General.lvlib\\Standby"(w544, error in=w545) -> (error out=w550:errorcluster)
            n147 = shared-variable "myRIO\\Library_Steering.lvlib\\STOP_Steering"(w544, error in=w550) -> (error out=w549:errorcluster)
            n148 = shared-variable "myRIO\\Library_Swimbladder.lvlib\\STOP_Swimbladder"(w544, error in=w549) -> (error out=w548:errorcluster)
            n149 = shared-variable "myRIO\\Library_Sensors.lvlib\\STOP_LiveStream"(w544, error in=w548) -> (error out=w547:errorcluster)
            n150 = while {
              tunnel: [w553] -> w546
              tunnel: w547 -> [w555]
              stop <- w552 stop-if-true
              n151 = shared-variable "myRIO\\Library_General.lvlib\\Reached Standby"(error in=w555) -> (w552:bool, error out=w554:errorcluster)
              n152 = Wait (ms)(milliseconds to wait=u32 10) -> ()  [unwired: 1 out]
              n153 = Not(x=w552) -> (.not. x?=w551:bool)
              n154 = call "Wait for myRIO"("error in (no error)"=w554, "Enable"=w551) -> ("error out"=w553:errorcluster)  [unwired: 8 in, 1 out]
            }
          }
          event "STOP_LiveStream": Value Change {
            n155 = event-data() -> ("NewVal"=w559:bool)  [unwired: 1 in, 5 out]
            n156 = shared-variable "myRIO\\Library_Sensors.lvlib\\STOP_LiveStream"(w559, error in=w562) -> (error out=w558:errorcluster)
            n157 = case shown="True" w559 {
              tunnel: [Sepios_status."Filming" ("Sepios_Status") Sepios_status."Running" ("Sepios_Status")] -> w561
              tunnel: w558 -> [w563 w566]
              tunnel: [w563 w565] -> w557
              frame False {
              }
              frame True {
                n158 = shared-variable "myRIO\\Library_Steering.lvlib\\Library_CollisionDetection.lvlib\\Collision Detected"(FALSE ("Collision Detected"), error in=w566) -> (error out=w565:errorcluster)
              }
            }
            n159 = shared-variable "myRIO\\Library_General.lvlib\\Library_Status.lvlib\\Sepios_Status"(w561, error in=w557) -> (error out=w560:errorcluster)
          }
          event "Collision\nAvoidance": Value Change {
            n160 = event-data() -> ("NewVal"=w570:bool)  [unwired: 1 in, 5 out]
            n161 = Not(x=w570) -> (.not. x?=w569:bool)
            n162 = shared-variable "myRIO\\Library_Steering.lvlib\\Library_CollisionDetection.lvlib\\STOP_CollisionAvoidance"(w569, error in=w572) -> (error out=w571:errorcluster)
            n163 = case shown="False" w570 {
              tunnel: w571 -> [w576 w577]
              tunnel: [w575 w577] -> w573
              frame False {
                n164 = shared-variable "myRIO\\Library_Steering.lvlib\\Library_CollisionDetection.lvlib\\Collision Detected"(FALSE ("Collision Detected"), error in=w576) -> (error out=w575:errorcluster)
              }
              frame True {
              }
            }
          }
          event "Collision\nDetection": Value Change {
            n165 = event-data() -> ("NewVal"=w580:bool)  [unwired: 1 in, 5 out]
            n166 = case shown="False" w580 {
              selector: w580 -> [w581 _]
              tunnel: w579 -> [w583 w584]
              tunnel: [w582 w584] -> w578
              frame False {
                n167 = property on="Collision\nAvoidance" class="Bool (strict)"(error in=w583, "Val(Sgnl)"=w581) -> (error out=w582:errorcluster)  [unwired: 1 in, 1 out]
              }
              frame True {
              }
            }
          }
          event "Full Battery?": Value Change {
            n168 = event-data() -> ("NewVal"=w588:bool)  [unwired: 1 in, 5 out]
            n169 = shared-variable "myRIO\\Library_General.lvlib\\Library_Status.lvlib\\Battrery_Full"(w588, error in=w589) -> (error out=w586:errorcluster)
            n170 = property on="Full Battery?" class="Bool (strict)"(error in=w586, "Value"=FALSE ("Full Battery?")) -> (error out=w585:errorcluster)  [unwired: 1 in, 1 out]
          }
          event "Exit": Value Change {
            n171 = event-data() -> ("NewVal"=w591:bool)  [unwired: 1 in, 5 out]
            n172 = shared-variable "myRIO\\Library_General.lvlib\\Exit"(w591, error in=w595) -> (error out=w596:errorcluster)
            n173 = shared-variable "myRIO\\Library_General.lvlib\\Standby"(w591, error in=w596) -> (error out=w598:errorcluster)
            n174 = shared-variable "myRIO\\Library_Steering.lvlib\\STOP_Steering"(w591, error in=w598) -> (error out=w597:errorcluster)
            n175 = shared-variable "myRIO\\Library_Swimbladder.lvlib\\STOP_Swimbladder"(w591, error in=w597) -> (error out=w593:errorcluster)
            n176 = shared-variable "myRIO\\Library_Steering.lvlib\\Library_CollisionDetection.lvlib\\STOP_CollisionAvoidance"(w591, error in=w593) -> (error out=w592:errorcluster)
            n177 = shared-variable "myRIO\\Library_Sensors.lvlib\\STOP_LiveStream"(w591, error in=w592) -> (error out=w590:errorcluster)
            n178 = shared-variable "myRIO\\Library_Log.lvlib\\STOP_Log"(w591, error in=w590) -> (error out=w594:errorcluster)
          }
          event "Save Parameters to File": Value Change {
            n179 = event-data() -> ()  [unwired: 1 in, 6 out]
            n180 = Get Date/Time String() -> (date string=w603:string)  [unwired: 3 in, 1 out]
            n181 = call <vilib>:"Application Directory.vi"() -> ("Application Directory"=w601:path)
            n182 = Concatenate Strings("Sepios Configuration " ("default name"), w603) -> (w600:string)
            n183 = call "File Dialog"("start path"=w601, "default name"=w600, "error in"=w599) -> ("selected path"=w607:path, "cancelled"=w606:bool, "error out"=w605:errorcluster)  [unwired: 9 in, 1 out]
            n184 = case shown="False" w606 {
              tunnel: w607 -> [w615 _]
              tunnel: w605 -> [w608 w617]
              tunnel: [w614 w617] -> w604
              frame False {
                n185 = invoke class="VI" method="Ctrl Val.Get All"(error in=w608, "Controls"=TRUE) -> (reference out=w611:refnum<vi>, error out=w610:errorcluster, "Get All Control Values Variant"=w612:cluster{"Name":string, "Variant Data":variant}[])  [unwired: 2 in, 1 out]
                n186 = Close Reference(reference=w611, error in (no error)=w610) -> (error out=w609:errorcluster)
                n187 = Flatten To XML(anything=w612) -> (xml string=w616:string)
                n188 = call-poly <vilib>:"Write to XML File.vi"("error in (no error)"=w609, "XML Input"=w616, "XML File Path"=w615) -> ("error out"=w614:errorcluster)  [unwired: 6 in, 2 out]
              }
              frame True {
              }
            }
          }
          event "Load Parameters from File": Value Change {
            n189 = event-data() -> ()  [unwired: 1 in, 6 out]
            n190 = Get Date/Time String() -> (date string=w621:string)  [unwired: 3 in, 1 out]
            n191 = call <vilib>:"Application Directory.vi"() -> ("Application Directory"=w619:path)
            n192 = Concatenate Strings("Sepios Configuration " ("default name"), w621) -> (w620:string)
            n193 = call "File Dialog2"("start path"=w619, "default name"=w620, "error in"=w618) -> ("selected path"=w626:path, "cancelled"=w625:bool, "error out"=w624:errorcluster)  [unwired: 9 in, 1 out]
            n194 = case shown="False" w625 {
              tunnel: w626 -> [w635 _]
              tunnel: w624 -> [w634 w636]
              tunnel: [w628 w636] -> w623
              frame False {
                n195 = call-poly <vilib>:"Read From XML File.vi"("error in (no error)"=w634, "XML File Path"=w635) -> ("error out"=w630:errorcluster, "XML Elements"=w633:string)  [unwired: 7 in, 1 out]
                n196 = Unflatten From XML(xml string=w633, type=cluster{"Name":string, "Variant Data":variant}[] [] ("Control Value:Get All"), error in (no error)=w630) -> (value=w632:cluster{"Name":string, "Variant Data":variant}[], error out=w629:errorcluster)
                n197 = Current VI's Path() -> (path=w631:path)
                n198 = call "Write_Control_Values.vi"("error in (no error)"=w629, "Path of VI with Controls to change"=w631, "Control Value:Get All 2"=w632) -> ("error out"=w628:errorcluster)  [unwired: 8 in]
              }
              frame True {
              }
            }
          }
          event "STOP_Swimbladder": Value Change {
            n199 = event-data() -> ("NewVal"=w640:bool)  [unwired: 1 in, 5 out]
            n200 = shared-variable "myRIO\\Library_Swimbladder.lvlib\\STOP_Swimbladder"(w640, error in=w637) -> (error out=w639:errorcluster)
            n201 = Wait (ms)(milliseconds to wait=u32 500) -> ()  [unwired: 1 out]
          }
          event "STOP_Steering": Value Change {
            # "#todo: Check variable"
            n202 = event-data() -> ("NewVal"=w643:bool)  [unwired: 1 in, 5 out]
            n203 = shared-variable "myRIO\\Library_Steering.lvlib\\STOP_Steering"(w643, error in=w641) -> (error out=w642:errorcluster)
          }
          event Value Change {
            n204 = event-data() -> ("NewVal"=w646:T28)  [unwired: 1 in, 5 out]
            n205 = shared-variable "myRIO\\Library_Sensors.lvlib\\Sensors State"(w646, error in=w644) -> (error out=w645:errorcluster)
          }
          event "Max Depth": Value Change {
            n206 = event-data() -> ("NewVal"=w647:dbl)  [unwired: 1 in, 5 out]
            n207 = shared-variable "myRIO\\Library_Swimbladder.lvlib\\Max Depth"(w647, error in=w648) -> (error out=w649:errorcluster)
          }
          event "Depth Desired [m]": Value Change {
            n208 = event-data() -> ("NewVal"=w650:dbl)  [unwired: 1 in, 5 out]
            n209 = shared-variable "myRIO\\Library_Swimbladder.lvlib\\Depth Desired"(w650, error in=w651) -> (error out=w652:errorcluster)
          }
          event Value Change {
            n210 = event-data() -> ("NewVal"=w653:T15)  [unwired: 1 in, 5 out]
            n211 = shared-variable "myRIO\\Library_Steering.lvlib\\Library_AttitudeControl.lvlib\\Attitude Controllers Parameters"(w653, error in=w655) -> (error out=w654:errorcluster)
          }
          event Value Change {
            n212 = event-data() -> ("NewVal"=w658:T7)  [unwired: 1 in, 5 out]
            n213 = shared-variable "myRIO\\Library_Steering.lvlib\\Intuitive Steering User Control"(w658, error in=w656) -> (error out=w657:errorcluster)
          }
          event Value Change {
            n214 = event-data() -> ("NewVal"=w661:T7)  [unwired: 1 in, 5 out]
            n215 = shared-variable "myRIO\\Library_Steering.lvlib\\Library_AttitudeControl.lvlib\\Intuitive Steering Attitude Control"(w661, error in=w660) -> (error out=w659:errorcluster)
          }
          event "Camera": Value Change {
            n216 = event-data() -> ("NewVal"=w662:bool)  [unwired: 1 in, 5 out]
            n217 = shared-variable "myRIO\\Library_General.lvlib\\Library_Status.lvlib\\CameraOn"(w662, error in=w664) -> (error out=w663:errorcluster)
          }
          event "Laser": Value Change {
            n218 = event-data() -> ("NewVal"=w667:bool)  [unwired: 1 in, 5 out]
            n219 = shared-variable "myRIO\\Library_General.lvlib\\Library_Status.lvlib\\LaserOn"(w667, error in=w666) -> (error out=w665:errorcluster)
          }
          event Value Change {
            n220 = event-data() -> ("NewVal"=w670:T8)  [unwired: 1 in, 5 out]
            n221 = shared-variable "myRIO\\Library_Steering.lvlib\\IndividualSteering_f(x)_enum"(w670, error in=w669) -> (error out=w668:errorcluster)
          }
          event Value Change {
            n222 = event-data() -> ("NewVal"=w673:T27)  [unwired: 1 in, 5 out]
            n223 = shared-variable "myRIO\\Library_SpaceMouse.lvlib\\SpaceMouse_Parameters"(w673, error in=w671) -> (error out=w672:errorcluster)
          }
          event Value Change {
            n224 = event-data() -> ("NewVal"=w676:T2)  [unwired: 1 in, 5 out]
            n225 = shared-variable "myRIO\\Library_Steering.lvlib\\Fin Arrangement"(w676, error in=w674) -> (error out=w675:errorcluster)
          }
          event Value Change {
            n226 = event-data() -> ("NewVal"=w679:T11)  [unwired: 1 in, 5 out]
            n227 = shared-variable "myRIO\\Library_Swimbladder.lvlib\\Swimbladder Tuning Parameters"(w679, error in=w677) -> (error out=w678:errorcluster)
          }
          event Value Change {
            n228 = event-data() -> ("NewVal"=w680:T31)  [unwired: 1 in, 5 out]
            n229 = shared-variable "myRIO\\Library_General.lvlib\\Sepios General Parameters"(w680, error in=w681) -> (error out=w682:errorcluster)
          }
          event Value Change {
            n230 = event-data() -> ("NewVal"=w683:T3)  [unwired: 1 in, 5 out]
            n231 = shared-variable "myRIO\\Library_Steering.lvlib\\Steering Mode"(w683, error in=w684) -> (error out=w685:errorcluster)
          }
        }
        n232 = shared-variable "myRIO\\Library_General.lvlib\\Exit"(error in=w428) -> (w429:bool, error out=w426:errorcluster)
        "Flow_LED" <- "Velocity Control on"
      }
      n233 = while {
        stop <- w163 stop-if-true
        # "Live Stream Manager"
        n234 = shared-variable "myRIO\\Library_Sensors.lvlib\\STOP_LiveStream"() -> (w161:bool)  [unwired: 1 in, 1 out]
        n235 = case shown="False" w161 {
          frame False {
            w165 = FALSE ("Record Button")
            n236 = property on="Record Button" class="Bool (strict)"("Value"=w165) -> ()  [unwired: 2 in, 2 out]
            n237 = property on="Picture Button" class="Bool (strict)"("Value"=w165) -> ()  [unwired: 2 in, 2 out]
            n238 = while {
              shift-right: [w182] -> _
              shift-left: w165 -> [w184]
              shift-right: [w181] -> _
              shift-left: _ -> [w180]
              shift-right: [w169] -> _
              shift-left: TRUE ("Laser Detected") -> [w168]
              stop <- w185 stop-if-true
              # "make subvi for avi and tiff..."
              n239 = shared-variable "myRIO\\Library_Sensors.lvlib\\STOP_LiveStream"() -> (w179:bool)  [unwired: 1 in, 1 out]
              n240 = case shown="False" w179 {
                tunnel: ["Record Button" FALSE ("Record Button")] -> w182
                frame False {
                }
                frame True {
                }
              }
              n241 = call "Vision Acquisition"("Stop (F)"=w179) -> ("Image Out"=w178:T30, "Stopped"=w185:bool)  [unwired: 23 in, 2 out]
              n242 = Equal?(x=w182, y=w184) -> (x = y?=w183:bool)
              n243 = case shown="True" w183 {
                tunnel: w182 -> [w211 w236]
                tunnel: [w210 w232] -> w181
                tunnel: w180 -> [w209 w235]
                tunnel: w178 -> [w208 w234]
                tunnel: [w208 w233] -> w176
                frame False {
                  n244 = case shown="True" w211 {
                    tunnel: [w212 w229] -> w210
                    tunnel: w209 -> [w212 _]
                    frame False {
                      n245 = call "IMAQ AVI2 Close"("AVI Refnum"=w212) -> ()  [unwired: 10 in, 1 out]
                    }
                    frame True {
                      w226 = TRUE ("replace all? (F)")
                      # "#todo: Codec and Quality"
                      n246 = Get Date/Time In Seconds() -> (seconds since 1Jan1904=w215:timestamp)
                      n247 = Format Date/Time String(seconds (now)=w215) -> (date/time string=w216:string)  [unwired: 2 in]
                      n248 = Search and Replace String(replace all?=w226, input string=w216, search string=":", replace string="." ("replace string (\"\")")) -> (result string=w224:string, error out=w227:errorcluster)  [unwired: 4 in, 2 out]
                      n249 = call <vilib>:"Space Constant.vi"() -> ("String"=w223:string)
                      n250 = Search and Replace String(replace all?=w226, input string=w224, search string=w223, replace string="_" ("replace string (\"\")"), error in=w227) -> (result string=w225:string)  [unwired: 3 in, 3 out]
                      n251 = Concatenate Strings("AVI Name", "_" ("string"), w225, ".avi" ("string")) -> (w228:string)
                      n252 = Build Path(base path="Path", name or relative path=w228) -> (appended path=w213:path)
                      n253 = call "IMAQ AVI2 Create"("Codec"="FF Video Codec 1 (FFV1) (NI Vision)", "Frames Per Second"=u32 10, "AVI Path"=w213) -> ("AVI Refnum"=w229:T39)  [unwired: 7 in, 1 out]
                    }
                  }
                }
                frame True {
                  n254 = case shown="False" w236 {
                    tunnel: w235 -> [w238 w242]
                    tunnel: w234 -> [w237 w241]
                    tunnel: [w237 w240] -> w233
                    tunnel: [w238 w239] -> w232
                    frame False {
                    }
                    frame True {
                      n255 = call "IMAQ AVI2 Write Frame"("Image"=w241, "AVI Refnum"=w242) -> ("Image Out (duplicate)"=w240:T30, "AVI Refnum (duplicate)"=w239:T39)  [unwired: 7 in, 1 out]
                    }
                  }
                }
              }
              n256 = case shown="True" "Picture Button" {
                tunnel: w178 -> [_ w204]
                frame False {
                }
                frame True {
                  w201 = TRUE ("replace all? (F)")
                  # "subVI for date and hour"
                  n257 = Get Date/Time In Seconds() -> (seconds since 1Jan1904=w191:timestamp)
                  n258 = property on="Path" class="Path"() -> ("Value"=w190:path)  [unwired: 2 in, 2 out]
                  n259 = Format Date/Time String(seconds (now)=w191) -> (date/time string=w192:string)  [unwired: 2 in]
                  n260 = Search and Replace String(replace all?=w201, input string=w192, search string=":", replace string="." ("replace string (\"\")")) -> (result string=w199:string, error out=w202:errorcluster)  [unwired: 4 in, 2 out]
                  n261 = call <vilib>:"Space Constant.vi"() -> ("String"=w198:string)
                  n262 = Search and Replace String(replace all?=w201, input string=w199, search string=w198, replace string="_" ("replace string (\"\")"), error in=w202) -> (result string=w200:string)  [unwired: 3 in, 3 out]
                  n263 = Concatenate Strings("Pic Name", "_" ("string"), w200, ".tiff" ("string")) -> (w186:string)
                  n264 = Build Path(base path=w190, name or relative path=w186) -> (appended path=w189:path)
                  n265 = call-poly "IMAQ Write File 2"("TIFF Options"=T34 {"Rows Per Strip"=0, "Photometric"=1, "Compression Type"=0}, "File Path"=w189, "Image"=w204) -> ("error out"=w203:errorcluster)  [unwired: 7 in, 1 out]
                  n266 = property on="Picture Button" class="Bool (strict)"(error in=w203, "Value"=FALSE ("Down Button")) -> ()  [unwired: 1 in, 2 out]
                }
              }
              n267 = call "CollisionDetection_main.vi"("Image In"=w176, "Collision\nDetection"="Collision\nDetection", "Overlay"="Overlay", "Laser Detected Old"=w168) -> ("Collision Detected"=→"Collision":bool, "Image Out"=→"Live Stream":T30, "Distance to Wall (m)"=→"Distance [m]":dbl, "Perpendicular Distance to Wall (m)"=→"Perp. Distance [m]":dbl, "delta° (incident angle)"=→"Incident Angle [°]":dbl, "Laser Detected"=w169:bool, "Laser Detected Twice"=→"Laser Detected":bool)  [unwired: 4 in, 1 out]
            }
          }
          frame True {
            n268 = Wait (ms)(milliseconds to wait=u32 50) -> ()  [unwired: 1 out]
          }
        }
        n269 = shared-variable "myRIO\\Library_General.lvlib\\Exit"() -> (w163:bool)  [unwired: 1 in, 1 out]
        n270 = Wait (ms)(milliseconds to wait=u32 50) -> ()  [unwired: 1 out]
      }
      n271 = while {
        tunnel: [w387] -> w129
        tunnel: w114 -> [w360]
        shift-right: [w370] -> w126
        shift-left: w121 -> [w369]
        stop <- w409 stop-if-true
        # "Monitor Indicators @ 100 Hz"
        n272 = shared-variable "myRIO\\Library_Steering.lvlib\\Servo Position"(error in=w360) -> (w393:T40, error out=w372:errorcluster)
        n273 = shared-variable "myRIO\\Library_Sensors.lvlib\\Attitude in radians"(error in=w372) -> (w373:cluster{"Roll":dbl, "Pitch":dbl, "Yaw":dbl}, error out=w371:errorcluster)
        n274 = Wait (ms)(milliseconds to wait=u32 10) -> ()  [unwired: 1 out]
        n275 = call "Attitude Control Write.vi"("error in (no error)"=w371, "Attitude in radians"=w373, "Attitude Control Handle In"=w369) -> ("error out"=w348:errorcluster, "Attitude Control Handle Out"=w370:T35)  [unwired: 7 in]
        n276 = Index Array(array=w393, index (row)=0 ("index")) -> (element=w353:dbl[])  [unwired: 1 in]
        n277 = Index Array(array=w393, index (row)=1 ("index")) -> (element=w406:dbl[])  [unwired: 1 in]
        n278 = Index Array(array=w393, index (row)=2 ("index")) -> (element=w407:dbl[])  [unwired: 1 in]
        n279 = Index Array(array=w393, index (row)=3 ("index")) -> (element=w408:dbl[])  [unwired: 1 in]
        n280 = shared-variable "myRIO\\Library_Sensors.lvlib\\Est_Position [m]"(error in=w348) -> (→"Estimated Position":T14, error out=w347:errorcluster)
        n281 = shared-variable "myRIO\\Library_General.lvlib\\Library_Status.lvlib\\Sepios_Status"(error in=w347) -> (→"Sepios_Status":T6, error out=w351:errorcluster)
        n282 = shared-variable "myRIO\\Library_Sensors.lvlib\\Main_Current"(error in=w351) -> (→"Main_Current [A]":dbl, error out=w356:errorcluster)
        n283 = Bundle(0.0, 1.0, "Servo Position"=w353) -> (→"Top Fin (0)":cluster{dbl, dbl, "Servo Position":dbl[]})  [unwired: 1 in]
        n284 = Bundle(0.0, 1.0, "Servo Position"=w406) -> (→"Right Fin (1)":cluster{dbl, dbl, "Servo Position":dbl[]})  [unwired: 1 in]
        n285 = Bundle(0.0, 1.0, "Servo Position"=w407) -> (→"Bottom Fin (2)":cluster{dbl, dbl, "Servo Position":dbl[]})  [unwired: 1 in]
        n286 = Bundle(0.0, 1.0, "Servo Position"=w408) -> (→"Left Fin (3)":cluster{dbl, dbl, "Servo Position":dbl[]})  [unwired: 1 in]
        n287 = shared-variable "myRIO\\Library_General.lvlib\\Library_Status.lvlib\\Battery_time_left"(error in=w356) -> (→"Time left [min]":dbl, error out=w366:errorcluster)
        n288 = shared-variable "myRIO\\Library_General.lvlib\\Library_Status.lvlib\\Battery_Level"(error in=w366) -> (w362:dbl, error out=w364:errorcluster)
        "Battery_level" <- w362
        n289 = Less?(x=w362, y=10.0) -> (x < y?=w363:bool)
        n290 = case shown="True" w363 {
          tunnel: w364 -> [w415 w419]
          tunnel: [w414 w418] -> w358
          frame False {
            n291 = property on="Battery_level" class="Slide (strict)"(error in=w415, "Fill Color"=u32 55040) -> (error out=w414:errorcluster)  [unwired: 1 in, 1 out]
          }
          frame True {
            n292 = property on="Battery_level" class="Slide (strict)"(error in=w419, "Fill Color"=u32 16719872) -> (error out=w418:errorcluster)  [unwired: 1 in, 1 out]
          }
        }
        n293 = shared-variable "myRIO\\Library_Log.lvlib\\slowSampling"(error in=w358) -> (→"Sampling Frequ.\ntoo LOW":bool, error out=w357:errorcluster)
        n294 = shared-variable "myRIO\\Library_Sensors.lvlib\\Depth_m [m]"(error in=w357) -> (w382:dbl, error out=w385:errorcluster)
        n295 = shared-variable "myRIO\\Library_Swimbladder.lvlib\\Depth Desired"(error in=w385) -> (w383:dbl, error out=w386:errorcluster)
        n296 = shared-variable "myRIO\\Library_Swimbladder.lvlib\\Max Depth"(error in=w386) -> (w384:dbl, error out=w374:errorcluster)
        n297 = Bundle("Double"=w382, "Double"=w383, w384) -> (→"Depth [m]":cluster{"Double":dbl, "Double":dbl, dbl})  [unwired: 1 in]
        n298 = shared-variable "myRIO\\Library_Swimbladder.lvlib\\X_desired"(error in=w374) -> (→"X_Desired":dbl, error out=w375:errorcluster)
        n299 = shared-variable "myRIO\\Library_Swimbladder.lvlib\\Advanced Swimbladder Indicators"(error in=w375) -> (w368:T12, error out=w378:errorcluster)
        "Advanced Swimbladder Indicators" <- w368
        n300 = shared-variable "myRIO\\Library_Sensors.lvlib\\IMU_Data_simple"(error in=w378) -> (→"IMU_Data_simple":T29, error out=w343:errorcluster)
        n301 = shared-variable "myRIO\\Library_Sensors.lvlib\\Flow_variables"(error in=w343) -> (→"Flow_variables":T41, error out=w344:errorcluster)
        n302 = shared-variable "myRIO\\Library_Steering.lvlib\\Brake"(error in=w344) -> (→"Brake":bool, error out=w346:errorcluster)
        n303 = shared-variable "myRIO\\Library_Steering.lvlib\\Library_CollisionDetection.lvlib\\Collision Detected"(error in=w346) -> (→"Avoidance":bool, error out=w345:errorcluster)
        n304 = shared-variable "myRIO\\Library_Steering.lvlib\\Fin Status"(error in=w345) -> (→"Fin Status":T1, error out=w355:errorcluster)
        n305 = disable-structure shown="Disabled" {
          disable-tunnel: w355 -> [w412 w413]
          disable-tunnel: [w411 w413] -> w354
          frame Disabled {
            n306 = shared-variable "myRIO\\Library_Steering.lvlib\\STOP_Steering"(error in=w412) -> (w410:bool, error out=w411:errorcluster)
            n307 = property on="STOP_Steering" class="Bool (strict)"("Value"=w410) -> ()  [unwired: 2 in, 2 out]
          }
          frame Enabled {
          }
        }
        n308 = shared-variable "myRIO\\Library_General.lvlib\\Exit"(error in=w354) -> (w409:bool, error out=w387:errorcluster)
        n309 = Unbundle By Name(w368) -> ("X_Actual [m]"=→"X_Actual [m]":dbl)
      }
      n310 = while {
        stop <- w245 stop-if-true
        # "#Todo: besser!"
        # "Space Mouse"
        n311 = Wait (ms)(milliseconds to wait=u32 50) -> ()  [unwired: 1 out]
        n312 = call "SpaceMouse_main.vi"() -> ()  [unwired: 12 in]
        n313 = disable-structure shown="Disabled" {
          frame Disabled {
            n314 = event shown="[0] \"SpaceMouse_Refresh\": Value Change" {
              selector: _ -> [_]
              dyn-events: _ -> [_]
              timeout: _ -> [_]
              event "SpaceMouse_Refresh": Value Change {
                n315 = event-data() -> ()  [unwired: 1 in, 4 out]
                n316 = property on="SpaceMouse_Refresh" class="Bool (strict)"("Value"=FALSE ("SpaceMouse_Refresh")) -> ()  [unwired: 2 in, 2 out]
              }
            }
          }
          frame Enabled {
          }
        }
        n317 = shared-variable "myRIO\\Library_General.lvlib\\Exit"() -> (w245:bool)  [unwired: 1 in, 1 out]
      }
      n318 = while {
        tunnel: w114 -> [w320]
        tunnel: [w317] -> w123
        stop <- w319 stop-if-true
        # "Graphen direkt in cluster integrieren, for loop!"
        # "Will be replaced by error \"loop\""
        n319 = shared-variable "myRIO\\Library_General.lvlib\\Library_Status.lvlib\\LeakageDetected"(error in=w320) -> (w324:bool, error out=w325:errorcluster)
        "LEAKAGE" <- w324
        n320 = case shown="False" w324 {
          tunnel: [w327 w334] -> w326
          tunnel: w325 -> [w327 w329]
          frame False {
          }
          frame True {
            n321 = call <vilib>:"Application Directory.vi"() -> ("Application Directory"=w331:path)
            n322 = Build Path(base path=w331, name or relative path="My Computer\\LeakageInterface\\RedAlert.wav") -> (appended path=w332:path)
            n323 = call <vilib>:"Play Sound File.vi"("timeout (sec)"=5000.0, "error in (no error)"=w329, "path"=w332, "device ID"=u32 0) -> ("error out"=w334:errorcluster)  [unwired: 6 in, 1 out]
          }
        }
        n324 = shared-variable "myRIO\\Library_General.lvlib\\Library_Status.lvlib\\tooDeep"(error in=w326) -> (w323:bool, error out=w321:errorcluster)
        "tooDeep" <- w323
        n325 = case shown="False" w323 {
          tunnel: w321 -> [w335 w340]
          tunnel: [w335 w337] -> w322
          frame False {
          }
          frame True {
            n326 = shared-variable "myRIO\\Library_Swimbladder.lvlib\\Depth Desired"(error in=w340) -> (w339:dbl, error out=w338:errorcluster)
            n327 = Negate(x=w339) -> (-x=w336:dbl)
            n328 = property on="Depth Desired [m]" class="DigNum (strict)"(error in=w338, "Value"=w336) -> (error out=w337:errorcluster)  [unwired: 1 in, 1 out]
          }
        }
        n329 = call "Display Message to User"("error in (no error)"=w322, "Enable"=w323) -> ("error out"=w316:errorcluster)  [unwired: 8 in, 1 out]
        n330 = shared-variable "myRIO\\Library_General.lvlib\\Library_Status.lvlib\\SB_Piston_Stuck"(error in=w316) -> (→"SB_Piston_Stuck":bool, error out=w315:errorcluster)
        n331 = shared-variable "myRIO\\Library_General.lvlib\\Exit"(error in=w315) -> (w319:bool, error out=w317:errorcluster)
        n332 = Wait (ms)(milliseconds to wait=u32 50) -> ()  [unwired: 1 out]
      }
      n333 = while {
        tunnel: [w152] -> w125
        tunnel: w115 -> [w155]
        tunnel: w114 -> [w154]
        stop <- w153 stop-if-true
        # "Log Main"
        n334 = call "Sensors_TDMS_write.vi"("TDMS: file name"="TDMS: file name", "Viewer_enable"="Viewer_enable", "base path"=w155, "Period [ms]"="Period [ms]", "group name"="group name", "channel name(s)"="channel name(s)", "error in"=w154) -> ("error out"=w150:errorcluster)  [unwired: 8 in]
        n335 = property on="Create New Log" class="Bool (strict)"(error in=w150, "Val(Sgnl)"=FALSE ("Value (Signaling)")) -> (error out=w149:errorcluster)  [unwired: 1 in, 1 out]
        n336 = shared-variable "myRIO\\Library_General.lvlib\\Exit"(error in=w149) -> (w153:bool, error out=w152:errorcluster)
      }
      n337 = call "Kalman_Estimator_Sepios.vi"("error in"=w114) -> ("error out"=w124:errorcluster)  [unwired: 10 in]
      n338 = call "battery.vi"("error IO in"=w114) -> ("error IO"=w117:errorcluster)  [unwired: 2 in]
      n339 = call "ErrorHandler.vi"("Error In"=w114, "base path"=w115) -> ("Error Out"=w116:errorcluster)  [unwired: 9 in]
      n340 = disable-structure shown="Disabled" {
        disable-tunnel: w114 -> [w131 w148]
        disable-tunnel: [w130 w148] -> w113
        frame Disabled {
          n341 = while {
            tunnel: w131 -> [w140]
            tunnel: [w147] -> w130
            shift-right: [w142] -> _
            shift-left: _ -> [w144]
            stop <- w146 stop-if-true
            n342 = Tick Count (ms)() -> (millisecond timer value=w143:u32)
            n343 = shared-variable "myRIO\\Library_Sensors.lvlib\\Flow_Speed"(error in=w140) -> (w141:dbl, error out=w137:errorcluster)
            "Speed [m/s]" <- w141
            "Value" <- w141
            "Speed" <- w141
            n344 = Wait (ms)(milliseconds to wait=u32 10) -> ()  [unwired: 1 out]
            n345 = To Double Precision Float(number=w143) -> (double precision float=w142:dbl)
            n346 = Subtract(x=w142, y=w144) -> (x-y=w145:dbl)
            n347 = Divide(x=w141, y=w145) -> (x/y=w139:dbl)
            n348 = Absolute Value(x=w139) -> (abs(x)=→"Acceleration [m/s2]":dbl)
            n349 = call "CalcDesiredVelVector_SpaceMouse_Input.vi"("error in (no error)"=w137, "Desired Speed(Throttle)"="Throttle") -> ("error IO"=w134:errorcluster)  [unwired: 9 in]
            n350 = call "Flow_spiderplot.vi"("error in"=w134) -> ("error out"=w133:errorcluster, "new picture"=→"spiderplot":picture)  [unwired: 4 in]
            n351 = shared-variable "myRIO\\Library_General.lvlib\\Exit"(error in=w133) -> (w146:bool, error out=w147:errorcluster)
          }
        }
        frame Enabled {
        }
      }
      n352 = Merge Errors(w113, w116, w117, w123, w124, w125, w129, w128) -> (w127:errorcluster)
    }
  }
  n353 = call "Attitude Control Close.vi"("error in (no error)"=w7, "Attitude Control Handle"=w5) -> ("error out"=w6:errorcluster)  [unwired: 9 in]
  n354 = call "Attitude Control Close.vi"("error in (no error)"=w6, "Attitude Control Handle"=w9) -> ("error out"=→"error out":errorcluster)  [unwired: 9 in]
